vi "main_INA231.vi"() -> ()   [LabVIEW 2011]
uses:
  <vilib>/Utility/file.llb/Read From Spreadsheet File (string).vi
  Global 1.vi
  <vilib>/Utility/file.llb/Write To Spreadsheet File (string).vi
  <vilib>/Utility/file.llb/Write To Spreadsheet File (DBL).vi
panel:
  out "Initial Time":dbl caption="Present (s)"
  out "Selected Path":path
  out "Power History":dbl[](array[numeric])
  out "Current History":dbl[](array[numeric])
  out "Shunt Voltage History":dbl[](array[numeric])
  out "Bus Voltage History":dbl[](array[numeric])
  in  "SM-DIG INT Voltage":enum16{"+3.3V", "+5V"}(ring)
  out "Shunt Voltage":dbl format="%#_4pV"
  out "Bus Voltage":dbl format="%#_4pV"
  out "Power":dbl format="%#_4pW"
  out "Current":dbl format="%#_4pA"
  out "Alert":bool
  out "Conv Ready Flag":bool
  in  "Power":bool=TRUE
  in  "Auto-Write":bool=TRUE
  out "Progress":u8(slide) scale=0.0..100.0
  out "Status":string
  in  "Write All Reg":bool
  in  "Read All Reg":bool
  out "Pending changes \nneed to be written":bool
  in  "Tab Control":T1(tab)
  in  "Enter Current LSB":dbl format="%#_4pA"
  out "High LSB":dbl format="%#_4pA"
  out "Low LSB":dbl format="%#_4pA"
  in  "Config Method":enum16{"Current LSB", "Calibration Register"}(ring)=enum."Calibration Register"
  in  "Enter Value for \nCalibration Register":u16
  in  "Enter Rshunt \nVariables":cluster{"Max Current":dbl, "Resistance":dbl} {"Resistance" format="%#_4p"; "Max Current" format="%#_4pA"}
  in  "Alert Limit":dbl min=0.0 max=0.0 format="%#_4pV"
  in  "Alert Config":T2(ring)=enum."None"
  in  "Conversion Ready":bool
  in  "Shunt Voltage Conversion Time":T3(ring)=enum."1.1ms"
  in  "Bus Voltage Conversion Time":T3(ring)=enum."1.1ms"
  in  "Operating Mode":T4(ring)=enum."Shunt and Bus, Continuous"
  in  "Averaging Mode":T5(ring)
  out "I2C Address":u8 format="%02x"
  in  "A1":u8(ring) items=["GND", "VS+", "SDA", "SCL"]
  in  "A0":u8(ring) items=["GND", "VS+", "SDA", "SCL"]
  out "Shunt Voltage":dbl format="%#_4pV"
  out "Bus Voltage":dbl format="%#_4pV"
  out "Power":dbl format="%#_4pW"
  out "Current":dbl format="%#_4pA"
  out "Current LSB":dbl format="%#_4pA"
  out "Rshunt (Ohms)":dbl format="%#_4p"
  out "Calibration":u16
  out "Shunt Voltage Bin":i16
  out "Current Bin":i16
  out "Power Bin":u16
  out "Bus Voltage Bin":u16
  out "Waveform Graph":dbl[](graph)
  in  "Continuously Poll Data":bool=TRUE
  in  "Graph Config":T6(ring)=enum."Vshunt (V)"
  in  "Help w Reg":bool
  in  "Register Table":i32(listbox)
  in  "dig_bits 16":T7 {"D15" max=1; "D14" max=1; "D13" max=1; "D12" max=1; "D11" max=1; "D10" max=1; "D9" max=1; "D8" max=1 format="%b"; "D7" max=1; "D6" max=1; "D5" max=1; "D4" max=1; "D3" max=1; "D2" max=1; "D1" max=1; "D0" max=1}
  in  "dig_bits8":T8 {"D7" max=1; "D6" max=1; "D5" max=1; "D4" max=1; "D3" max=1; "D2" max=1; "D1" max=1; "D0" max=1}
  out "Bit_Config_16b.csv":path
  out "Start USB DAQ":path
  out "Table_Config.csv":path
  out "USB DAQ INI":path
  out "SAve USB Config":path
  out "Calculate":bool
  out "USB DAQ Vref":dbl min=0.0 max=5.0
  out "USB DAQ Address":i32 format="%x"
  out "DAC Mode":i32
  out "ADS Mode":i32
  out "USB DAQ Vsup":dbl min=0.0 max=5.0
  in  "Register":u16[](array[numeric]) format="%x"
  out "bit_text_array":string[][](array[string])=[["d0", "d1", "d2", "d3", "d4", "d5", "d6", "d7"], ["a0", "a1", "a2", "a3", "a4", "a5", "a6", "a7"]]
  out "Digital out":u16
  out "Reg_Numb":i32
  out "Number of Registers":i32
  in  "PORT2":i16=152 format="%x"
  out "Numb_Bits_In_Reg":i32=16
  out "Edited Register":bool[](array[boolean])
  out "Index to Reg No":u8[](array[numeric]) format="%x"
  out "Alert Limit Digital":i16
  in  "Write I2C Address":u8 format="%x"
  out "RAR trigger":bool
  out "1st Time?":bool
  # "Step 4: Select Configuration Method"
  # "Step 5: Set Configuration Register"
  # "Current LSB"
  # "Step 6: Configure Alert Pin"
  # "Step 3: Set Conversion Times"
  # "Bus Conversion"
  # "Shunt Conversion"
  # "Step 2: Configure Operation"
  # "Step 1: Set I2C Address"
  # "This tab gives a flow chart of how the calculations within the INA226 occur"
  # "Current * Bus Voltage"
  # "__________________"
  # "Power ="
  # "20000"
  # "Shunt Voltage * Cal"
  # "________________"
  # "Current ="
  # "2048"
  # ".00512"
  # "_________________"
  # "Cal ="
  # "Current LSB *Rshunt"
  # "20000"
  # "÷"
  # "2048"
  # "÷"
  # ".00512"
  # "÷"
  # "X"
  # "X"
  # "X"
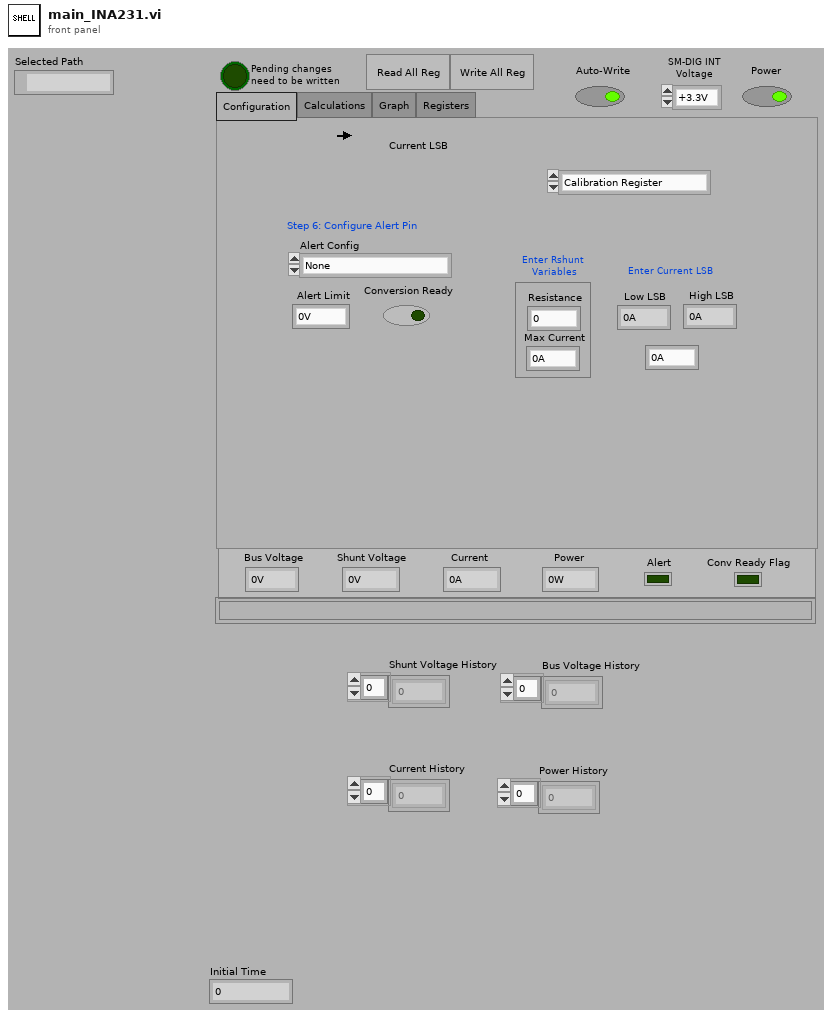
[diagram p1: front panel]
types:
  T1 = enum32{"Configuration", "Calculations", "Graph", "Registers", "Debug", "Internal Variables"}
  T2 = enum16{"Over-Limit Power", "Bus Voltage Under-Voltage", "Bus Voltage Over-Voltage", "Shunt Voltage Under-Voltage", "Shunt Voltage Over-Voltage", "None"}
  T3 = enum16{"140us", "204us", "332us", "588us", "1.1ms", "2.116ms", "4.156ms", "8.244ms"}
  T4 = enum16{"Power Down", "Shunt Voltage, Triggered", "Bus Voltage, Triggered", "Shunt and Bus, Triggered", "Power Down ", "Shunt Voltage, Continuous", "Bus Voltage, Continuous", "Shunt and Bus, Continuous"}
  T5 = enum16{"1", "4", "16", "64", "128", "256", "512", "1024"}
  T6 = enum16{"Vbus (V)", "Vshunt (V)", "Current (A)", "Power (W)"}
  T7 = cluster{"D0":u16, "D1":u16, "D2":u16, "D3":u16, "D4":u16, "D5":u16, "D6":u16, "D7":u16, "D8":u16, "D9":u16, "D10":u16, "D11":u16, "D12":u16, "D13":u16, "D14":u16, "D15":u16}
  T8 = cluster{"D0":u16, "D1":u16, "D2":u16, "D3":u16, "D4":u16, "D5":u16, "D6":u16, "D7":u16}
  T9 = enum16{"Always On", "Always Off", "Off While Running"}
  T10 = enum32{"Invalid", "Standard", "Closed", "Hidden", "Minimized", "Maximized"}
  T11 = enum16{"Over-Limit Power", "Bus Voltage Under-Voltage", "Bus Voltage Over-Voltage", "Shunt Voltage Under-Voltage", "Shunt Voltage Over-Voltage"}
  T12 = enum32{"invalid app kind", "Development System", "Run Time System", "Student Edition", "Embedded LabVIEW", "Evaluation", "Custom"}
  T13 = typedef "LVRowAndColumnTypeDef.ctl" = cluster{"Row":i32, "Column":i32}
  T14 = cluster{"[0]":u16, "[1]":u16, "[2]":u16, "[3]":u16, "[4]":u16, "[5]":u16, "[6]":u16, "[7]":u16}
  T15 = cluster{"[0]":u16, "[1]":u16, "[2]":u16, "[3]":u16, "[4]":u16, "[5]":u16, "[6]":u16, "[7]":u16, "[8]":u16, "[9]":u16, "[10]":u16, "[11]":u16, "[12]":u16, "[13]":u16, "[14]":u16, "[15]":u16}
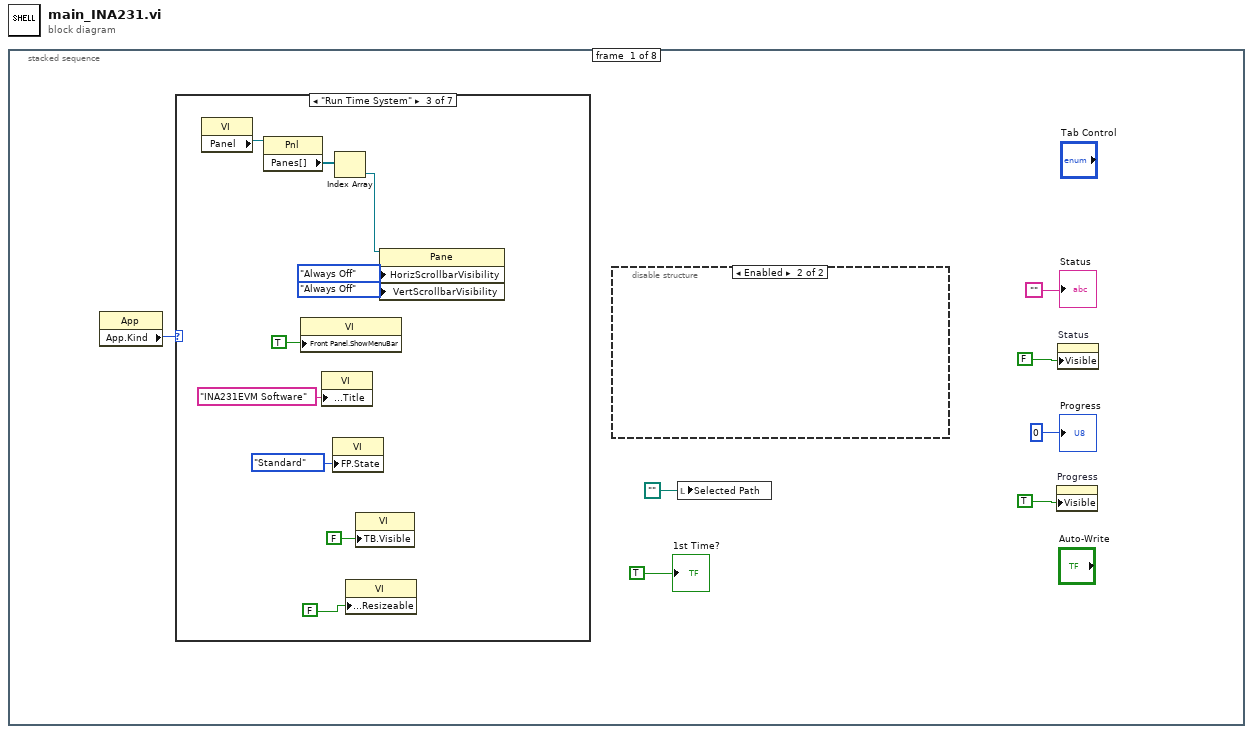
[diagram p0: block diagram]
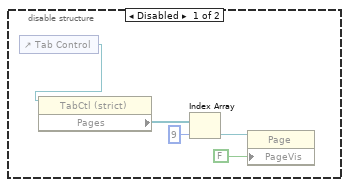
[diagram p2: hidden frame]
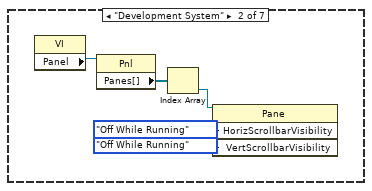
[diagram p4: hidden frame]
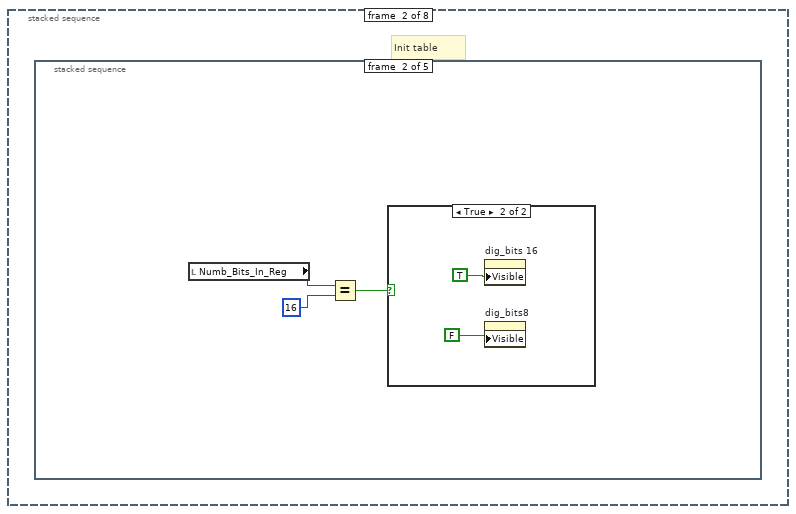
[diagram p9: hidden frame]
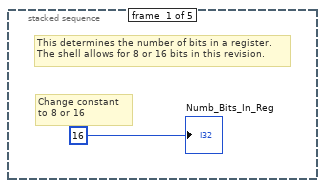
[diagram p10: hidden frame]
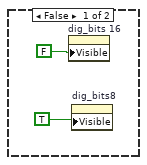
[diagram p11: hidden frame]
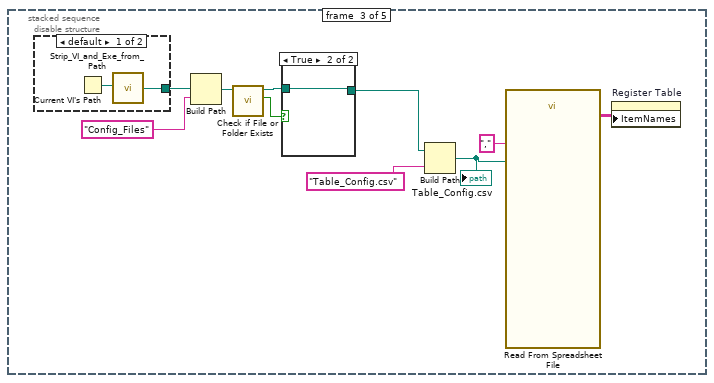
[diagram p12: hidden frame]
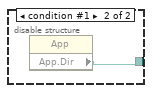
[diagram p13: hidden frame]
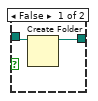
[diagram p14: hidden frame]
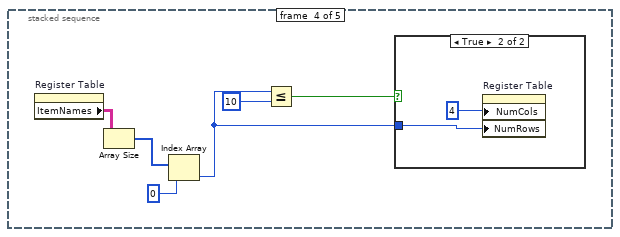
[diagram p15: hidden frame]
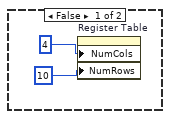
[diagram p16: hidden frame]
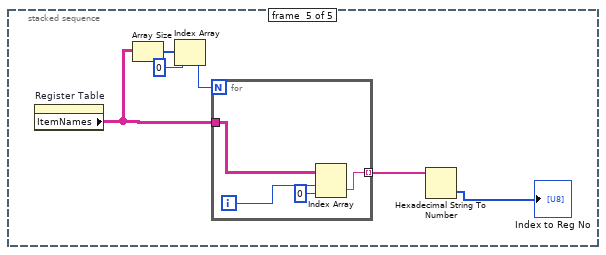
[diagram p17: hidden frame]
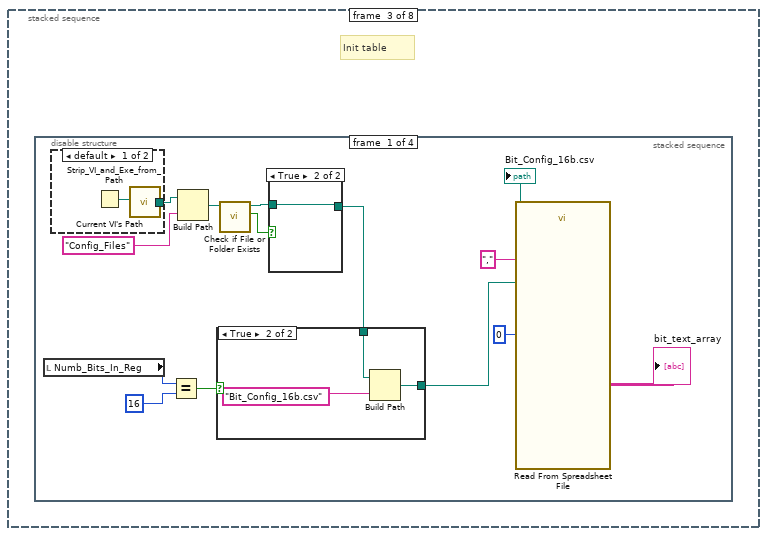
[diagram p18: hidden frame]
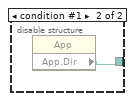
[diagram p19: hidden frame]
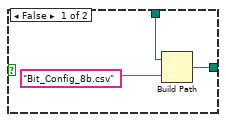
[diagram p20: hidden frame]
diagram:
  n1 = stacked-sequence {
    frame #0 {
      n2 = property class="App"() -> ("App.Kind"=w7:T12)  [unwired: 2 in, 2 out]
      n3 = case shown="\"Run Time System\"" w7 {
        frame "invalid app kind", Default {
        }
        frame "Development System" {
          n4 = property class="VI"() -> ("Panel"=w17:refnum<vi>)  [unwired: 2 in, 2 out]
          n5 = property class="Pnl"(reference=w17) -> ("Panes[]"=w16:refnum<vi>[])  [unwired: 1 in, 2 out]
          n6 = Index Array(array=w16) -> (element=w15:refnum<vi>)  [unwired: 1 in]
          n7 = property class="Pane"(reference=w15, "HorizScrollbarVisibility"=T9."Off While Running" ("Horizontal Scrollbar Visibility"), "VertScrollbarVisibility"=T9."Off While Running" ("Vertical Scrollbar Visibility")) -> ()  [unwired: 1 in, 2 out]
        }
        frame "Run Time System" {
          n8 = property class="VI"() -> ("Panel"=w27:refnum<vi>)  [unwired: 2 in, 2 out]
          n9 = property class="Pnl"(reference=w27) -> ("Panes[]"=w26:refnum<vi>[])  [unwired: 1 in, 2 out]
          n10 = property class="VI"("Front Panel.ShowMenuBar"=TRUE ("Front Panel Window:Show Menu Bar")) -> ()  [unwired: 2 in, 2 out]
          n11 = property class="VI"("Front Panel.Title"="INA231EVM Software" ("Front Panel Window:Title")) -> ()  [unwired: 2 in, 2 out]
          n12 = property class="VI"("FP.State"=T10."Standard" ("Front Panel Window:State")) -> ()  [unwired: 2 in, 2 out]
          n13 = Index Array(array=w26) -> (element=w25:refnum<vi>)  [unwired: 1 in]
          n14 = property class="VI"("Front Panel.Resizeable"=FALSE ("Front Panel Window:Resizeable")) -> ()  [unwired: 2 in, 2 out]
          n15 = property class="VI"("TB.Visible"=FALSE ("Front Panel Window:Resizeable")) -> ()  [unwired: 2 in, 2 out]
          n16 = property class="Pane"(reference=w25, "HorizScrollbarVisibility"=T9."Always Off" ("Horizontal Scrollbar Visibility"), "VertScrollbarVisibility"=T9."Always Off" ("Vertical Scrollbar Visibility")) -> ()  [unwired: 1 in, 2 out]
        }
        frame "Student Edition" {
        }
        frame "Embedded LabVIEW" {
        }
        frame "Evaluation" {
        }
        frame "Custom" {
        }
      }
      n17 = disable-structure shown="Enabled" {
        frame Disabled {
          n18 = control-ref of="Tab Control"() -> (w8:refnum<vi>)
          n19 = property class="TabCtl (strict)"(reference=w8) -> ("Pages"=w11:refnum<vi>[])  [unwired: 1 in, 2 out]
          n20 = Index Array(array=w11, index=9) -> (element=w9:refnum<vi>)
          n21 = property class="Page"(reference=w9, "PageVis"=FALSE ("Page Visible")) -> ()  [unwired: 1 in, 2 out]
        }
        frame Enabled {
        }
      }
      n22 = local write "Selected Path"(path "") -> ()
      n23 = property on="Progress" class="Slide (strict)"("Visible"=TRUE ("Front Panel Window:Resizeable")) -> ()  [unwired: 2 in, 2 out]
      n24 = property on="Status" class="Str"("Visible"=FALSE ("Front Panel Window:Resizeable")) -> ()  [unwired: 2 in, 2 out]
      "Progress" <- u8 0 ("Progress")
      "Status" <- ""
      "1st Time?" <- TRUE ("1st Time?")
    }
    frame #1 {
      # "Init table"
      n25 = stacked-sequence {
        frame #0 {
          # "Change constant \nto 8 or 16"
          # "This determines the number of bits in a register.\nThe shell allows for 8 or 16 bits in this revision."
          "Numb_Bits_In_Reg" <- 16
        }
        frame #1 {
          n26 = local read "Numb_Bits_In_Reg"() -> (w31:i32)
          n27 = Equal?(x=w31, y=16) -> (x = y?=w30:bool)
          n28 = case shown="True" w30 {
            frame False {
              n29 = property on="dig_bits 16" class="Clust (strict)"("Visible"=FALSE) -> ()  [unwired: 2 in, 2 out]
              n30 = property on="dig_bits8" class="Clust (strict)"("Visible"=TRUE) -> ()  [unwired: 2 in, 2 out]
            }
            frame True {
              n31 = property on="dig_bits 16" class="Clust (strict)"("Visible"=TRUE) -> ()  [unwired: 2 in, 2 out]
              n32 = property on="dig_bits8" class="Clust (strict)"("Visible"=FALSE) -> ()  [unwired: 2 in, 2 out]
            }
          }
        }
        frame #2 {
          n33 = disable-structure shown="default" {
            disable-tunnel: [w46 w48] -> w44
            frame condition #0 (active) {
              n34 = Current VI's Path() -> (path=w47:path)
              n35 = call "Strip_VI_and_Exe_from_Path.vi"("App Path"=w47) -> ("App Path out"=w46:path)
            }
            frame condition #1 {
              n36 = property class="App"() -> ("App.Dir"=w48:path)  [unwired: 2 in, 2 out]
            }
          }
          n37 = Build Path(base path=w44, name or relative path="Config_Files" ("path name")) -> (appended path=w43:path)
          n38 = call <vilib>:"Check if File or Folder Exists.vi"("path"=w43) -> ("file or folder exists?"=w42:bool, "dup path"=w41:path)  [unwired: 8 in, 1 out]
          n39 = case shown="True" w42 {
            tunnel: w41 -> [w50 w51]
            tunnel: [w49 w51] -> w38
            frame False {
              n40 = Create Folder(path (use dialog)=w50) -> (created path=w49:path)  [unwired: 2 in, 2 out]
            }
            frame True {
            }
          }
          n41 = Build Path(base path=w38, name or relative path="Table_Config.csv") -> (appended path=w45:path)
          "Table_Config.csv" <- w45
          n42 = call-poly <vilib>:"Read From Spreadsheet File.vi"("delimiter (\\t)"="," ("delimiter (\\t)"), "file path (dialog if empty)"=w45) -> ("all rows"=w37:string[][])  [unwired: 5 in, 4 out]
          n43 = property on="Register Table" class="MCListbox (strict)"("ItemNames"=w37) -> ()  [unwired: 2 in, 2 out]
        }
        frame #3 {
          n44 = property on="Register Table" class="MCListbox (strict)"() -> ("ItemNames"=w52:string[][])  [unwired: 2 in, 2 out]
          n45 = Array Size(array=w52) -> (size(s)=w53:i32[])
          n46 = Index Array(array=w53, index=0) -> (element=w57:i32)
          n47 = Less Or Equal?(x=w57, y=10) -> (x <= y?=w55:bool)
          n48 = case shown="True" w55 {
            tunnel: w57 -> [_ w60]
            frame False {
              n49 = property on="Register Table" class="MCListbox (strict)"("NumCols"=u32 4 ("Number of Columns"), "NumRows"=u32 10 ("Number of Rows")) -> ()  [unwired: 2 in, 2 out]
            }
            frame True {
              n50 = property on="Register Table" class="MCListbox (strict)"("NumCols"=u32 4 ("Number of Columns"), "NumRows"=w60) -> ()  [unwired: 2 in, 2 out]
            }
          }
        }
        frame #4 {
          n51 = property on="Register Table" class="MCListbox (strict)"() -> ("ItemNames"=w63:string[][])  [unwired: 2 in, 2 out]
          n52 = Array Size(array=w63) -> (size(s)=w65:i32[])
          n53 = Index Array(array=w65, index=0) -> (element=w67:i32)
          n54 = for {
            N: w67 -> [_]
            tunnel: w63 -> [w70]
            tunnel: [w68] -> w64 mode=indexing
            i -> [w71]
            n55 = Index Array(array=w70, index (row)=w71, index (col)=0 ("disabled index (col)")) -> (element=w68:string)
          }
          n56 = Hexadecimal String To Number(string=w64) -> (number=→"Index to Reg No":u32[])  [unwired: 2 in, 1 out]
        }
      }
    }
    frame #2 {
      # "Init table"
      n57 = stacked-sequence {
        frame #0 {
          n58 = local read "Numb_Bits_In_Reg"() -> (w74:i32)
          n59 = disable-structure shown="default" {
            disable-tunnel: [w85 w87] -> w72
            frame condition #0 (active) {
              n60 = Current VI's Path() -> (path=w86:path)
              n61 = call "Strip_VI_and_Exe_from_Path.vi"("App Path"=w86) -> ("App Path out"=w85:path)
            }
            frame condition #1 {
              n62 = property class="App"() -> ("App.Dir"=w87:path)  [unwired: 2 in, 2 out]
            }
          }
          n63 = Equal?(x=w74, y=16) -> (x = y?=w75:bool)
          n64 = Build Path(base path=w72, name or relative path="Config_Files" ("path name")) -> (appended path=w83:path)
          n65 = call <vilib>:"Check if File or Folder Exists.vi"("path"=w83) -> ("file or folder exists?"=w82:bool, "dup path"=w81:path)  [unwired: 8 in, 1 out]
          n66 = case shown="True" w82 {
            tunnel: w81 -> [w95 w96]
            tunnel: [w94 w96] -> w79
            frame False {
              n67 = Create Folder(path (use dialog)=w95) -> (created path=w94:path)  [unwired: 2 in, 2 out]
            }
            frame True {
            }
          }
          n68 = case shown="True" w75 {
            tunnel: [w88 w93] -> w84
            tunnel: w79 -> [w89 w91]
            frame False {
              n69 = Build Path(base path=w89, name or relative path="Bit_Config_8b.csv") -> (appended path=w88:path)
            }
            frame True {
              n70 = Build Path(base path=w91, name or relative path="Bit_Config_16b.csv") -> (appended path=w93:path)
            }
          }
          "Bit_Config_16b.csv" <- w84
          n71 = call-poly <vilib>:"Read From Spreadsheet File.vi"("delimiter (\\t)"="," ("delimiter (\\t)"), "start of read offset (chars.:0)"=0, "file path (dialog if empty)"=w84) -> ("all rows"=→"bit_text_array":string[][])  [unwired: 4 in, 4 out]
        }
        frame #1 {
          n72 = property on="Register Table" class="MCListbox (strict)"() -> ("ItemNames"=w104:string[][])  [unwired: 2 in, 2 out]
          n73 = local read "bit_text_array"() -> (w99:string[][])
          n74 = Array Size(array=w104) -> (size(s)=w103:i32[])
          n75 = Index Array(array=w103, index=0) -> (element=w105:i32)
          n76 = Array Size(array=w99) -> (size(s)=w98:i32[])
          n77 = Index Array(array=w98, index=0) -> (element=w97:i32)
          n78 = Not Equal?(x=w105, y=w97) -> (x != y?=w101:bool)
          n79 = case shown="True" w101 {
            frame False {
            }
            frame True {
              n80 = One Button Dialog(message="The number of rows in \"Bit_Config.csv\"  is not \nequal to the number of rows in \"Table_Config.csv\"" ("button name (\"OK\")")) -> ()  [unwired: 1 in, 1 out]
            }
          }
        }
        frame #2 {
          # "init table rows and col"
          n81 = property on="Register Table" class="MCListbox (strict)"("ColHdrString"=string[] ["Addr", "Name", "Status", "Hex", "Value"] ("Column Header Strings[]")) -> ()  [unwired: 2 in, 2 out]
        }
        frame #3 {
          n82 = local write "Pending changes \nneed to be written"(FALSE ("Pending changes \nneed to be written")) -> ()
          n83 = local read "bit_text_array"() -> (w115:string[][])
          n84 = Array Size(array=w115) -> (size(s)=w114:i32[])
          n85 = Index Array(array=w114, index=0) -> (element=w109:i32)
          "Number of Registers" <- w109
          n86 = Initialize Array(FALSE ("Boolean"), w109) -> (→"Edited Register":bool[])
          n87 = Initialize Array(0 ("element"), w109) -> (w108:i32[])
          n88 = local write "Register"(w108) -> ()
          n89 = disable-structure shown="Disabled" {
            frame Disabled {
              n90 = property on="Register" class="Arr (strict)" props=["Val(Sgnl)"]() -> ()  [unwired: 3 in, 2 out]
            }
            frame Enabled {
            }
          }
        }
      }
    }
    frame #3 {
      n91 = Current VI's Path() -> (path=w122:path)
      n92 = call "Load_USB_DAQ_Config_File.vi"("App Path"=w122) -> ("USB DAQ Vsup"=→"USB DAQ Vsup":dbl, "USB DAQ Address"=→"USB DAQ Address":i32, "DAC Mode"=→"DAC Mode":i32, "ADS Mode"=→"ADS Mode":i32, "USB DAQ Vref"=→"USB DAQ Vref":dbl)
    }
    frame #4 {
      n93 = flat-sequence {
        frame #0 {
          n94 = call "TI_INIT.vi"() -> ()  [unwired: 1 in, 2 out]
        }
        frame #1 {
          n95 = local read "USB DAQ Address"() -> (w126:i32)
          n96 = Current VI's Path() -> (path=w125:path)
          "Start USB DAQ" <- w125
          n97 = call "Start_USB_DAQ.vi"("USB ADDRESS In"=w126, "App Path"=w125) -> ("Abort"=w124:bool, "USB ADDRESS 0ut"=w123:i32)
          n98 = local write "USB DAQ Address"(w123) -> ()
          n99 = Stop(stop? (T)=w124) -> ()
        }
        frame #2 {
          # "Power on for typical starting conditions"
          n100 = local read "USB DAQ Address"() -> (w128:i32)
          n101 = local write "PORT2"(i16 152 ("PORT2")) -> ()
          n102 = call "VDUT ON.vi"("Device address"=w128) -> ()  [unwired: 2 in, 1 out]
        }
      }
    }
    frame #5 {
      w132 = dbl[] [] ("History Data")
      w141 = 0.0 ("Power")
      w146 = 0.0 ("Power")
      w140 = FALSE
      n103 = local read "Enter Rshunt \nVariables"() -> (w142:cluster{"Max Current":dbl, "Resistance":dbl})
      n104 = local write "I2C Address"(w141) -> ()
      n105 = Bundle By Name(cluster=w142, "Max Current"=w141, "Resistance"=w141) -> (w143:cluster{"Max Current":dbl, "Resistance":dbl})
      n106 = local write "Enter Rshunt \nVariables"(w143) -> ()
      n107 = local write "Config Method"(enum16{"Current LSB", "Calibration Register"}."Current LSB" ("Config Method")) -> ()
      n108 = local write "Operating Mode"(T4."Shunt Voltage, Continuous" ("Operating Mode")) -> ()
      n109 = local write "Shunt Voltage Conversion Time"(T3."1.1ms" ("Shunt Voltage Conversion Time")) -> ()
      n110 = local write "Bus Voltage Conversion Time"(T3."1.1ms" ("Bus Voltage Conversion Time")) -> ()
      n111 = local write "Alert Config"(T2."None" ("Alert Config")) -> ()
      n112 = local write "Alert Limit"(w141) -> ()
      n113 = local write "A0"(w141) -> ()
      n114 = local write "Write I2C Address"(u8 128 ("Write I2C Address")) -> ()
      n115 = local write "A1"(w141) -> ()
      n116 = local write "Averaging Mode"(w141) -> ()
      n117 = local write "Enter Value for \nCalibration Register"(w146) -> ()
      n118 = local write "Enter Current LSB"(w146) -> ()
      n119 = local write "High LSB"(w146) -> ()
      n120 = local write "Low LSB"(w146) -> ()
      n121 = local write "Shunt Voltage"(w146) -> ()
      n122 = local write "Continuously Poll Data"(w140) -> ()
      n123 = local write "Current"(w146) -> ()
      n124 = local write "Conversion Ready"(w140) -> ()
      n125 = local write "Bus Voltage"(w146) -> ()
      n126 = local write "Alert"(w140) -> ()
      n127 = local write "Conv Ready Flag"(w140) -> ()
      n128 = local write "Power"(w146) -> ()
      n129 = local write "Graph Config"(T6."Vbus (V)" ("Graph Config")) -> ()
      n130 = global read "Global 1.vi" "SAve USB Config"() -> (→"SAve USB Config":path)
      n131 = global read "Global 1.vi" "USB DAQ INI"() -> (→"USB DAQ INI":path)
      n132 = property on="Enter Value for \nCalibration Register" class="DigNum (strict)"("Visible"=FALSE) -> ()  [unwired: 2 in, 2 out]
      n133 = property on="Max Current" class="DigNum (strict)"("Visible"=TRUE) -> ()  [unwired: 2 in, 2 out]
      n134 = property on="Enter Current LSB" class="DigNum (strict)"("Visible"=TRUE) -> ()  [unwired: 2 in, 2 out]
      n135 = property on="Low LSB" class="DigNum (strict)"("Visible"=TRUE) -> ()  [unwired: 2 in, 2 out]
      n136 = property on="High LSB" class="DigNum (strict)"("Visible"=TRUE) -> ()  [unwired: 2 in, 2 out]
      n137 = local write "Shunt Voltage History"(w132) -> ()
      n138 = local write "Current History"(w132) -> ()
      n139 = local write "Bus Voltage History"(w132) -> ()
      n140 = local write "Power History"(w132) -> ()
      n141 = local write "Waveform Graph"(w132) -> ()
    }
    frame #6 {
      n142 = property on="RAR trigger" class="Bool (strict)"("Val(Sgnl)"=TRUE) -> ()  [unwired: 2 in, 2 out]
    }
    frame #7 {
      n143 = while {
        stop <- w151 stop-if-true
        n144 = event shown="[2] Menu Selection (User)" {
          selector: _ -> [_ _ _ _ _ _ _ _ _ _ _ _ _ _ _ _ _ _ _ _ _ _ _ _ _ _ _ _ _]
          dyn-events: _ -> [_ _ _ _ _ _ _ _ _ _ _ _ _ _ _ _ _ _ _ _ _ _ _ _ _ _ _ _ _]
          timeout: 800 -> [_ _ _ _ _ _ _ _ _ _ _ _ _ _ _ _ _ _ _ _ _ _ _ _ _ _ _ _ _]
          tunnel: [_ _ _ w233 _ _ _ _ _ _ _ _ _ _ _ _ _ _ _ _ _ _ _ _ _ _ _ _ _] -> w151
          event Timeout {
            n145 = event-data() -> ()  [unwired: 1 in, 2 out]
            n146 = case shown="True" "Continuously Poll Data" {
              frame False {
                n147 = property on="Write All Reg" class="Bool"() -> ("Disabled"=w153:u8)  [unwired: 2 in, 2 out]
                n148 = case shown="0, Default" w153 {
                  frame 0, Default {
                  }
                  frame 1 {
                  }
                  frame 2 {
                    n149 = property on="Write All Reg" class="Bool"("Disabled"=u8 0) -> ()  [unwired: 2 in, 2 out]
                  }
                }
              }
              frame True {
                n150 = stacked-sequence {
                  frame #0 {
                    n151 = local read "1st Time?"() -> (w155:bool)
                    n152 = case shown="True" w155 {
                      frame False {
                      }
                      frame True {
                        n153 = call "Elapsed Time"() -> ("Present (s)"=w157:dbl)  [unwired: 12 in, 7 out]
                        n154 = local write "Initial Time"(w157) -> ()
                        n155 = local write "1st Time?"(FALSE ("1st Time?")) -> ()
                      }
                    }
                  }
                  frame #1 {
                    n156 = property on="Write All Reg" class="Bool"("Disabled"=u8 2) -> ()  [unwired: 2 in, 2 out]
                    n157 = property on="RAR trigger" class="Bool (strict)"("Val(Sgnl)"=TRUE) -> ()  [unwired: 2 in, 2 out]
                  }
                }
              }
            }
          }
          event "Graph Config": Value Change {
            n158 = event-data() -> ()  [unwired: 1 in, 6 out]
            n159 = case shown="\"Current (A)\"" "Graph Config" {
              frame "Vbus (V)", Default {
                n160 = local read "Bus Voltage History"() -> (w161:dbl[])
                n161 = local write "Waveform Graph"(w161) -> ()
              }
              frame "Vshunt (V)" {
                n162 = local read "Shunt Voltage History"() -> (w162:dbl[])
                n163 = local write "Waveform Graph"(w162) -> ()
              }
              frame "Current (A)" {
                n164 = local read "Current History"() -> (w163:dbl[])
                n165 = local write "Waveform Graph"(w163) -> ()
              }
              frame "Power (W)" {
                n166 = local read "Power History"() -> (w164:dbl[])
                n167 = local write "Waveform Graph"(w164) -> ()
              }
            }
          }
          event Menu Selection (User) {
            n168 = event-data() -> ("MenuRef"=w165:refnum<k9>, "ItemTag"=w166:string)  [unwired: 1 in, 5 out]
            n169 = stacked-sequence {
              tunnel: w166 -> [w169 w173 w178 w183 w186 _]
              tunnel: w166 -> [_ _ _ _ _ w216]
              tunnel: w165 -> [_ _ _ _ w185 _]
              frame #0 {
                n170 = Equal?(x=w169, y="Control / Measure Bits") -> (x = y?=w168:bool)
                n171 = case shown="True" w168 {
                  frame False {
                  }
                  frame True {
                    n172 = local read "USB DAQ Address"() -> (w170:i32)
                    n173 = call "GPIO_Control.vi"("Device address"=w170) -> ()
                  }
                }
              }
              frame #1 {
                n174 = Equal?(x=w173, y="DAC / ADC Control") -> (x = y?=w171:bool)
                n175 = case shown="True" w171 {
                  frame False {
                  }
                  frame True {
                    n176 = local read "USB DAQ Address"() -> (w174:i32)
                    n177 = local read "ADS Mode"() -> (w176:i32)
                    n178 = call "ADC_and_DAC.vi"("ADS Mode In"=w176, "Board address"=w174) -> ("ADS Mode Out"=w175:i32)
                    n179 = local write "ADS Mode"(w175) -> ()
                  }
                }
              }
              frame #2 {
                n180 = Equal?(x=w178, y="Run Mnemonic Commands") -> (x = y?=w179:bool)
                n181 = case shown="True" w179 {
                  frame False {
                  }
                  frame True {
                    n182 = local read "USB DAQ Address"() -> (w180:i32)
                    n183 = call "Run_4_Cmds.vi"("USB DAQ Address"=w180) -> ()  [unwired: 2 in]
                  }
                }
              }
              frame #3 {
                n184 = Equal?(x=w183, y="Debug") -> (x = y?=w181:bool)
                n185 = case shown="False" w181 {
                  frame False {
                  }
                  frame True {
                    n186 = call "TI_Debug_Window.vi"() -> ()  [unwired: 1 in]
                  }
                }
              }
              frame #4 {
                w184 = "Make All Visible" ("y")
                n187 = Equal?(x=w186, y=w184) -> (x = y?=w187:bool)
                n188 = case shown="True" w187 {
                  tunnel: w185 -> [_ w189]
                  tunnel: w184 -> [_ w190]
                  frame False {
                  }
                  frame True {
                    n189 = Get Menu Item Info(7:w190, 11:w189) -> (3:w188:refnum<k9>, 4:w191:bool)  [unwired: 1 in, 5 out]
                    n190 = case shown="False" w191 {
                      tunnel: w190 -> [w193 w205]
                      tunnel: w188 -> [w192 w204]
                      frame True {
                        n191 = stacked-sequence {
                          tunnel: w193 -> [_ _ w202]
                          tunnel: w192 -> [_ _ w201]
                          frame #0 {
                            n192 = control-ref of="Tab Control"() -> (w194:refnum<vi>)
                            n193 = property class="TabCtl (strict)"(reference=w194) -> ("Pages"=w197:refnum<vi>[])  [unwired: 1 in, 2 out]
                            n194 = Index Array(array=w197, index=4) -> (element=w195:refnum<vi>)
                            n195 = property class="Page"(reference=w195, "PageVis"=FALSE ("Page Visible")) -> ()  [unwired: 1 in, 2 out]
                          }
                          frame #1 {
                            n196 = property on="Status" class="Str"("Visible"=TRUE ("Page Visible")) -> ()  [unwired: 2 in, 2 out]
                            n197 = property on="Progress" class="Slide (strict)"("Visible"=TRUE) -> ()  [unwired: 2 in, 2 out]
                          }
                          frame #2 {
                            n198 = Set Menu Item Info(6:FALSE ("checked"), 7:w202, 11:w201) -> ()  [unwired: 4 in, 2 out]
                          }
                        }
                      }
                      frame False {
                        n199 = stacked-sequence {
                          tunnel: w205 -> [_ _ w214]
                          tunnel: w204 -> [_ _ w213]
                          frame #0 {
                            n200 = control-ref of="Tab Control"() -> (w206:refnum<vi>)
                            n201 = property class="TabCtl (strict)"(reference=w206) -> ("Pages"=w209:refnum<vi>[])  [unwired: 1 in, 2 out]
                            n202 = Index Array(array=w209, index=4) -> (element=w207:refnum<vi>)
                            n203 = property class="Page"(reference=w207, "PageVis"=TRUE ("Page Visible")) -> ()  [unwired: 1 in, 2 out]
                          }
                          frame #1 {
                            n204 = property on="Status" class="Str"("Visible"=TRUE ("Page Visible")) -> ()  [unwired: 2 in, 2 out]
                            n205 = property on="Progress" class="Slide (strict)"("Visible"=TRUE) -> ()  [unwired: 2 in, 2 out]
                          }
                          frame #2 {
                            n206 = Set Menu Item Info(6:TRUE ("checked"), 7:w214, 11:w213) -> ()  [unwired: 4 in, 2 out]
                          }
                        }
                      }
                    }
                  }
                }
              }
              frame #5 {
                n207 = Equal?(x=w216, y="Start Graph Log") -> (x = y?=w217:bool)
                n208 = case shown="True" w217 {
                  frame False {
                  }
                  frame True {
                    n209 = Current VI's Path() -> (path=w226:path)
                    n210 = call "Open_File_from_Folder.vi"("path name"="Output Data", "prompt"="Save Config File", "pattern label"="CSV File ", "pattern (all files)"="*.csv", "App Path"=w226) -> ("selected path"=w220:path, "cancelled"=w221:bool)
                    n211 = local write "1st Time?"(TRUE ("1st Time?")) -> ()
                    n212 = case shown="False" w221 {
                      tunnel: w220 -> [w227 _]
                      frame False {
                        n213 = call-poly <vilib>:"Write To Spreadsheet File.vi"("delimiter (\\t)"="," ("delimiter (\\t)"), "append to file? (new file:F)"=TRUE, "1D data"=string[] ["Time", "Vbus", "Vshunt", "Current", "Power"], "file path (dialog if empty)"=w227) -> ()  [unwired: 4 in, 1 out]
                        "Selected Path" <- w227
                      }
                      frame True {
                        n214 = local write "Selected Path"(path "") -> ()
                      }
                    }
                  }
                }
              }
            }
          }
          event Panel Close? {
            n215 = event-data() -> ()  [unwired: 1 in, 4 out]
            n216 = flat-sequence {
              tunnel: [w237] -> w232
              tunnel: [w239] -> w233
              tunnel: w232 -> [w239]
              frame #0 {
                n217 = Two Button Dialog(message="Are you sure that you want to close this application?", 1:"No" ("F button name (\"Cancel\")"), 2:"Yes" ("T button name (\"OK\")")) -> (T button?=w237:bool)
              }
              frame #1 {
                n218 = case shown="True" w239 {
                  frame False {
                  }
                  frame True {
                    n219 = call "tio32_Close.vi"() -> ()  [unwired: 6 in, 3 out]
                  }
                }
              }
            }
            n220 = Not(x=w233) -> (.not. x?=w234:bool)
            n221 = event-data("Discard?"=w234) -> ()  [unwired: 1 in, 1 out]
          }
          event "SM-DIG INT Voltage": Value Change {
            n222 = event-data() -> ()  [unwired: 1 in, 6 out]
            n223 = case shown="\"+3.3V\", Default" "SM-DIG INT Voltage" {
              frame "+3.3V", Default {
                n224 = local read "PORT2"() -> (w241:i16)
                n225 = call "SM_VDUT SEL.vi"("Port2 IN"=w241, "Power Voltage"=enum16{"+3.3V", "+5V"}."+3.3V") -> ("Port2 OUT"=w242:u8)  [unwired: 1 in, 1 out]
                n226 = local write "PORT2"(w242) -> ()
              }
              frame "+5V" {
                n227 = local read "PORT2"() -> (w244:i16)
                n228 = call "SM_VDUT SEL.vi"("Port2 IN"=w244, "Power Voltage"=enum16{"+3.3V", "+5V"}."+5V") -> ("Port2 OUT"=w245:u8)  [unwired: 1 in, 1 out]
                n229 = local write "PORT2"(w245) -> ()
              }
            }
          }
          event "dig_bits 16", "dig_bits8": Value Change {
            n230 = event-data() -> ()  [unwired: 1 in, 6 out]
            n231 = stacked-sequence {
              frame #0 {
                n232 = local write "Digital out"(u16 0 ("Digital out")) -> ()
              }
              frame #1 {
                # "Converts the cluster of bits to a decimal equivelant."
                n233 = local read "Numb_Bits_In_Reg"() -> (w251:i32)
                n234 = Equal?(x=w251, y=16) -> (x = y?=w249:bool)
                n235 = case shown="True" w249 {
                  tunnel: [w252 w255] -> w248
                  frame False {
                    n236 = Cluster To Array(cluster="dig_bits8") -> (array=w252:u16[])
                  }
                  frame True {
                    n237 = Cluster To Array(cluster="dig_bits 16") -> (array=w255:u16[])
                  }
                }
                n238 = for {
                  tunnel: w248 -> [w258] mode=indexing
                  i -> [w257]
                  n239 = local read "Digital out"() -> (w259:u16)
                  n240 = Logical Shift(y=w257, x=w258) -> (x << y=w260:u16)
                  n241 = Add(x=w260, y=w259) -> (x+y=→"Digital out":u16)
                }
              }
              frame #2 {
                # "Takes the decimal equivelant from the bit cluster and places\n it into the list box."
                n242 = local read "Numb_Bits_In_Reg"() -> (w266:i32)
                n243 = local read "Digital out"() -> (w269:u16)
                n244 = Number To Hexadecimal String(1:i16 2 ("width (-)"), 2:w269) -> (0:w263:string)
                n245 = local read "Reg_Numb"() -> (w271:i32)
                n246 = Equal?(x=w266, y=8) -> (x = y?=w264:bool)
                n247 = property on="Register Table" class="MCListbox (strict)"() -> ("ItemNames"=w268:string[][])  [unwired: 2 in, 2 out]
                n248 = case shown="False" w264 {
                  tunnel: w263 -> [w272 w274]
                  tunnel: [w272 w273] -> w262
                  frame False {
                  }
                  frame True {
                    n249 = String Subset(string=w274, length (rest)=2 ("length (rest)")) -> (substring=w273:string)  [unwired: 1 in]
                  }
                }
                n250 = Replace Array Subset(array=w268, new element=w262, index (row)=w271, index (col)=3 ("disabled index (col)")) -> (w267:string[][])
                n251 = property on="Register Table" class="MCListbox (strict)"("ItemNames"=w267) -> ()  [unwired: 2 in, 2 out]
              }
              frame #3 {
                # "Takes the decimal equivelant from the bit cluster and \nputs it into the \"Register\" array."
                n252 = local read "Reg_Numb"() -> (w277:i32)
                n253 = local read "Digital out"() -> (w279:u16)
                n254 = local read "Register"() -> (w278:u16[])
                n255 = Replace Array Subset(array=w278, new element=w279, index=w277) -> (w276:u16[])
                n256 = property on="Register" class="Arr (strict)"("Val(Sgnl)"=w276) -> ()  [unwired: 2 in, 2 out]
              }
              frame #4 {
                n257 = local read "Edited Register"() -> (w283:bool[])
                n258 = local read "Reg_Numb"() -> (w280:i32)
                n259 = Replace Array Subset(array=w283, new element=TRUE ("new element/subarray"), index=w280) -> (w281:bool[])
                n260 = property on="Edited Register" class="Arr (strict)"("Val(Sgnl)"=w281) -> ()  [unwired: 2 in, 2 out]
              }
            }
          }
          event "RAR trigger": Value Change; "Read All Reg": Mouse Up {
            n261 = event-data() -> ()  [unwired: 1 in, 4 out]
            n262 = stacked-sequence {
              frame #0 {
                n263 = property on="Status" class="Str"("Visible"=FALSE ("Front Panel Window:Resizeable")) -> ()  [unwired: 2 in, 2 out]
                n264 = property on="Progress" class="Slide (strict)"("Visible"=TRUE ("Front Panel Window:Resizeable")) -> ()  [unwired: 2 in, 2 out]
              }
              frame #1 {
                # "Call External \"Read All Reg\" VI"
                n265 = local read "USB DAQ Address"() -> (w290:i32)
                n266 = local read "Write I2C Address"() -> (w286:u8)
                n267 = local read "Register"() -> (w289:u16[])
                n268 = local read "Index to Reg No"() -> (w287:u8[])
                n269 = control-ref of="Progress"() -> (w291:refnum<vi>)
                n270 = call "Read_All_Reg.vi"("Register"=w289, "Slide Refnum"=w291, "USB DAQ Address"=w290, "Read I2C Address"=w286, "Index to Reg No"=w287) -> ("Output Register"=w292:u16[], "Status"=w288:string)
                n271 = property on="Register" class="Arr (strict)"("Val(Sgnl)"=w292) -> ()  [unwired: 2 in, 2 out]
                n272 = property on="Status" class="Str"("Val(Sgnl)"=w288) -> ()  [unwired: 2 in, 2 out]
              }
              frame #2 {
                # "Change status of registers to indicate that they have been written to"
                n273 = local read "Current History"() -> (w301:dbl[])
                n274 = local read "Shunt Voltage History"() -> (w303:dbl[])
                n275 = local read "Shunt Voltage"() -> (w304:dbl)
                n276 = local read "Current"() -> (w300:dbl)
                n277 = local read "Number of Registers"() -> (w308:i32)
                n278 = Insert Into Array(array=w303, new element=w304) -> (w302:dbl[])  [unwired: 1 in]
                n279 = Insert Into Array(array=w301, new element=w300) -> (w299:dbl[])  [unwired: 1 in]
                n280 = local write "Shunt Voltage History"(w302) -> ()
                n281 = local write "Current History"(w299) -> ()
                n282 = local write "Pending changes \nneed to be written"(FALSE ("Pending changes \nneed to be written")) -> ()
                n283 = Initialize Array(FALSE ("Boolean"), w308) -> (w306:bool[])
                n284 = local read "Bus Voltage History"() -> (w294:dbl[])
                n285 = local write "Edited Register"(w306) -> ()
                n286 = local read "Power History"() -> (w298:dbl[])
                n287 = local read "Bus Voltage"() -> (w295:dbl)
                n288 = local read "Power"() -> (w297:dbl)
                n289 = Insert Into Array(array=w294, new element=w295) -> (w293:dbl[])  [unwired: 1 in]
                n290 = Insert Into Array(array=w298, new element=w297) -> (w296:dbl[])  [unwired: 1 in]
                n291 = local write "Bus Voltage History"(w293) -> ()
                n292 = local write "Power History"(w296) -> ()
              }
              frame #3 {
                # "Remove all bold from table"
                n293 = local read "Number of Registers"() -> (w309:i32)
                n294 = for {
                  N: w309 -> [_]
                  i -> [w310]
                  n295 = for {
                    N: 4 -> [_]
                    tunnel: w310 -> [w312]
                    i -> [w313]
                    n296 = stacked-sequence {
                      tunnel: w313 -> [w317 _]
                      tunnel: w312 -> [w316 _]
                      frame #0 {
                        n297 = property on="Register Table" class="MCListbox (strict)"() -> ("ActiveCell"=w315:T13)  [unwired: 2 in, 2 out]
                        n298 = Bundle By Name(cluster=w315, "Row"=w316, "Column"=w317) -> (w314:T13)
                        n299 = property on="Register Table" class="MCListbox (strict)"("ActiveCell"=w314) -> ()  [unwired: 2 in, 2 out]
                      }
                      frame #1 {
                        n300 = property on="Register Table" class="MCListbox (strict)"("CellFontBold"=FALSE ("Active Cell:Cell Font:Bold")) -> ()  [unwired: 2 in, 2 out]
                      }
                    }
                  }
                }
              }
              frame #4 {
                # "Update the Calculate Tab"
                n301 = local read "Graph Config"() -> (w319:T6)
                n302 = case shown="\"Power (W)\"" w319 {
                  frame "Vbus (V)", Default {
                    n303 = local read "Bus Voltage History"() -> (w323:dbl[])
                    n304 = local write "Waveform Graph"(w323) -> ()
                  }
                  frame "Vshunt (V)" {
                    n305 = local read "Shunt Voltage History"() -> (w324:dbl[])
                    n306 = local write "Waveform Graph"(w324) -> ()
                  }
                  frame "Current (A)" {
                    n307 = local read "Current History"() -> (w325:dbl[])
                    n308 = local write "Waveform Graph"(w325) -> ()
                  }
                  frame "Power (W)" {
                    n309 = local read "Power History"() -> (w326:dbl[])
                    n310 = local write "Waveform Graph"(w326) -> ()
                  }
                }
                n311 = local read "Calculate"() -> (w321:bool)
                n312 = Exclusive Or(1:w321, 2:TRUE ("Calculate")) -> (0:w320:bool)
                n313 = property on="Calculate" class="Bool (strict)"("Val(Sgnl)"=w320) -> ()  [unwired: 2 in, 2 out]
              }
              frame #5 {
                n314 = local read "Selected Path"() -> (w327:path)
                n315 = Not Equal?(x=w327, y=path "") -> (x != y?=w328:bool)
                n316 = case shown="True" w328 {
                  tunnel: w327 -> [_ w337]
                  frame False {
                  }
                  frame True {
                    n317 = call "Elapsed Time"() -> ("Present (s)"=w339:dbl)  [unwired: 12 in, 7 out]
                    n318 = local read "Bus Voltage"() -> (w335:dbl)
                    n319 = local read "Shunt Voltage"() -> (w334:dbl)
                    n320 = local read "Current"() -> (w333:dbl)
                    n321 = local read "Power"() -> (w332:dbl)
                    n322 = local read "Initial Time"() -> (w338:dbl)
                    n323 = Subtract(x=w339, y=w338) -> (x-y=w336:dbl)
                    n324 = Build Array(w336, w335, w334, w333, w332) -> (w331:dbl[])
                    n325 = call-poly <vilib>:"Write To Spreadsheet File.vi"("delimiter (\\t)"="," ("delimiter (\\t)"), "format (%.3f)"="%#g", "append to file? (new file:F)"=TRUE, "1D data"=w331, "file path (dialog if empty)"=w337) -> ()  [unwired: 3 in, 1 out]
                  }
                }
              }
            }
          }
          event "Write All Reg": Mouse Up {
            n326 = event-data() -> ()  [unwired: 1 in, 8 out]
            n327 = stacked-sequence {
              frame #0 {
                n328 = local read "Operating Mode"() -> (w342:T4)
                n329 = property on="Status" class="Str"("Visible"=FALSE ("Front Panel Window:Resizeable")) -> ()  [unwired: 2 in, 2 out]
                n330 = property on="Progress" class="Slide (strict)"("Visible"=TRUE ("Front Panel Window:Resizeable")) -> ()  [unwired: 2 in, 2 out]
                n331 = case shown="\"Power Down \"" w342 {
                  frame "Power Down", Default {
                  }
                  frame "Shunt Voltage, Triggered" {
                    w347 = u16 0  # Reg Number
                    n332 = local read "Edited Register"() -> (w346:bool[])
                    n333 = Replace Array Subset(array=w346, new element=TRUE ("new element/subarray"), index=w347) -> (w345:bool[])
                    n334 = property on="Edited Register" class="Arr (strict)"("Val(Sgnl)"=w345) -> ()  [unwired: 2 in, 2 out]
                  }
                  frame "Bus Voltage, Triggered" {
                    w351 = u16 0  # Reg Number
                    n335 = local read "Edited Register"() -> (w350:bool[])
                    n336 = Replace Array Subset(array=w350, new element=TRUE ("new element/subarray"), index=w351) -> (w349:bool[])
                    n337 = property on="Edited Register" class="Arr (strict)"("Val(Sgnl)"=w349) -> ()  [unwired: 2 in, 2 out]
                  }
                  frame "Shunt and Bus, Triggered" {
                    w355 = u16 0  # Reg Number
                    n338 = local read "Edited Register"() -> (w354:bool[])
                    n339 = Replace Array Subset(array=w354, new element=TRUE ("new element/subarray"), index=w355) -> (w353:bool[])
                    n340 = property on="Edited Register" class="Arr (strict)"("Val(Sgnl)"=w353) -> ()  [unwired: 2 in, 2 out]
                  }
                  frame "Power Down " {
                  }
                  frame "Shunt Voltage, Continuous" {
                  }
                  frame "Bus Voltage, Continuous" {
                  }
                  frame "Shunt and Bus, Continuous" {
                  }
                }
              }
              frame #1 {
                # "Call external \"Write All Reg\" VI"
                n341 = local read "USB DAQ Address"() -> (w360:i32)
                n342 = local read "Edited Register"() -> (w363:bool[])
                n343 = control-ref of="Progress"() -> (w361:refnum<vi>)
                n344 = local read "Register"() -> (w362:u16[])
                n345 = local read "Index to Reg No"() -> (w357:u8[])
                n346 = call "Write_All_Reg.vi"("USB DAQ Address"=w360, "Write I2C Address"="Write I2C Address", "Edited Register"=w363, "Slide Refnum"=w361, "Index to Reg No"=w357, "Register"=w362) -> ("Status"=w358:string)
                n347 = property on="Status" class="Str"("Val(Sgnl)"=w358) -> ()  [unwired: 2 in, 2 out]
              }
              frame #2 {
                # "Change status of registers to indicate that they have been written to"
                n348 = local read "Number of Registers"() -> (w367:i32)
                n349 = local write "Pending changes \nneed to be written"(FALSE ("Pending changes \nneed to be written")) -> ()
                n350 = Initialize Array(FALSE ("Boolean"), w367) -> (w365:bool[])
                n351 = local write "Edited Register"(w365) -> ()
              }
              frame #3 {
                # "Remove all bold from table"
                n352 = local read "Number of Registers"() -> (w368:i32)
                n353 = for {
                  N: w368 -> [_]
                  i -> [w369]
                  n354 = for {
                    N: 4 -> [_]
                    tunnel: w369 -> [w371]
                    i -> [w372]
                    n355 = stacked-sequence {
                      tunnel: w372 -> [w376 _]
                      tunnel: w371 -> [w375 _]
                      frame #0 {
                        n356 = property on="Register Table" class="MCListbox (strict)"() -> ("ActiveCell"=w374:T13)  [unwired: 2 in, 2 out]
                        n357 = Bundle By Name(cluster=w374, "Row"=w375, "Column"=w376) -> (w373:T13)
                        n358 = property on="Register Table" class="MCListbox (strict)"("ActiveCell"=w373) -> ()  [unwired: 2 in, 2 out]
                      }
                      frame #1 {
                        n359 = property on="Register Table" class="MCListbox (strict)"("CellFontBold"=FALSE ("Active Cell:Cell Font:Bold")) -> ()  [unwired: 2 in, 2 out]
                      }
                    }
                  }
                }
              }
            }
          }
          event "Auto-Write": Value Change {
            n360 = event-data() -> ()  [unwired: 1 in, 6 out]
            n361 = local read "Auto-Write"() -> (w378:bool)
            n362 = case shown="True" w378 {
              frame False {
              }
              frame True {
                n363 = stacked-sequence {
                  frame #0 {
                    n364 = property on="Status" class="Str"("Visible"=FALSE ("Front Panel Window:Resizeable")) -> ()  [unwired: 2 in, 2 out]
                    n365 = property on="Progress" class="Slide (strict)"("Visible"=TRUE ("Front Panel Window:Resizeable")) -> ()  [unwired: 2 in, 2 out]
                  }
                  frame #1 {
                    # "Call external \"Write All Reg\" VI"
                    n366 = local read "Write I2C Address"() -> (w382:u8)
                    n367 = local read "USB DAQ Address"() -> (w384:i32)
                    n368 = local read "Edited Register"() -> (w387:bool[])
                    n369 = control-ref of="Progress"() -> (w385:refnum<vi>)
                    n370 = local read "Register"() -> (w386:u16[])
                    n371 = local read "Index to Reg No"() -> (w381:u8[])
                    n372 = call "Write_All_Reg.vi"("USB DAQ Address"=w384, "Write I2C Address"=w382, "Edited Register"=w387, "Slide Refnum"=w385, "Index to Reg No"=w381, "Register"=w386) -> ("Status"=w383:string)
                    n373 = property on="Status" class="Str"("Val(Sgnl)"=w383) -> ()  [unwired: 2 in, 2 out]
                  }
                  frame #2 {
                    # "Change status of registers to indicate that they have been written to"
                    n374 = local read "Number of Registers"() -> (w391:i32)
                    n375 = local write "Pending changes \nneed to be written"(FALSE ("Pending changes \nneed to be written")) -> ()
                    n376 = Initialize Array(FALSE ("Boolean"), w391) -> (w389:bool[])
                    n377 = local write "Edited Register"(w389) -> ()
                  }
                  frame #3 {
                    # "Remove all bold from table"
                    n378 = local read "Number of Registers"() -> (w392:i32)
                    n379 = for {
                      N: w392 -> [_]
                      i -> [w393]
                      n380 = for {
                        N: 4 -> [_]
                        tunnel: w393 -> [w395]
                        i -> [w396]
                        n381 = stacked-sequence {
                          tunnel: w396 -> [w400 _]
                          tunnel: w395 -> [w399 _]
                          frame #0 {
                            n382 = property on="Register Table" class="MCListbox (strict)"() -> ("ActiveCell"=w398:T13)  [unwired: 2 in, 2 out]
                            n383 = Bundle By Name(cluster=w398, "Row"=w399, "Column"=w400) -> (w397:T13)
                            n384 = property on="Register Table" class="MCListbox (strict)"("ActiveCell"=w397) -> ()  [unwired: 2 in, 2 out]
                          }
                          frame #1 {
                            n385 = property on="Register Table" class="MCListbox (strict)"("CellFontBold"=FALSE ("Active Cell:Cell Font:Bold")) -> ()  [unwired: 2 in, 2 out]
                          }
                        }
                      }
                    }
                  }
                }
              }
            }
          }
          event "A0": Value Change {
            # "A0 represents the 2nd and 3rd bit of the I2C Address\nSee Table 1 in the INA226 datatsheet for explanation"
            n386 = event-data() -> ()  [unwired: 1 in, 6 out]
            n387 = local read "Write I2C Address"() -> (w410:u8)
            n388 = Logical Shift(y=i8 1, x="A0") -> (x << y=w407:u8)
            n389 = And(x=u8 248 ("y"), y=w410) -> (x .and. y?=w408:u8)
            n390 = Or(x=w407, y=w408) -> (x .or. y?=w404:u8)
            n391 = local write "Write I2C Address"(w404) -> ()
            n392 = Logical Shift(y=i8 -1, x=w404) -> (x << y=w405:u8)
            n393 = local write "I2C Address"(w405) -> ()
          }
          event "A1": Value Change {
            # "A1 represents the 4th and 5th bit of the I2C Write Address\nSee Table 1 in the INA226 datatsheet for explanation"
            n394 = event-data() -> ()  [unwired: 1 in, 6 out]
            n395 = local read "Write I2C Address"() -> (w419:u8)
            n396 = Logical Shift(y=i8 3, x="A1") -> (x << y=w416:u8)
            n397 = And(x=u8 230 ("y"), y=w419) -> (x .and. y?=w417:u8)
            n398 = Or(x=w416, y=w417) -> (x .or. y?=w412:u8)
            n399 = local write "Write I2C Address"(w412) -> ()
            n400 = Logical Shift(y=i8 -1, x=w412) -> (x << y=→"I2C Address":u8)
          }
          event "Status": Value Change {
            n401 = event-data() -> ()  [unwired: 1 in, 6 out]
            n402 = local read "Status"() -> (w422:string)
            n403 = Equal?(x=w422, y="") -> (x = y?=w420:bool)
            n404 = case shown="True" w420 {
              frame False {
                n405 = property on="Status" class="Str"("Visible"=TRUE ("Front Panel Window:Resizeable")) -> ()  [unwired: 2 in, 2 out]
                n406 = property on="Progress" class="Slide (strict)"("Visible"=FALSE ("Front Panel Window:Resizeable")) -> ()  [unwired: 2 in, 2 out]
              }
              frame True {
                n407 = property on="Progress" class="Slide (strict)"("Visible"=TRUE ("Front Panel Window:Resizeable")) -> ()  [unwired: 2 in, 2 out]
                n408 = property on="Status" class="Str"("Visible"=FALSE ("Front Panel Window:Resizeable")) -> ()  [unwired: 2 in, 2 out]
              }
            }
          }
          event "Power": Mouse Up {
            n409 = event-data() -> ()  [unwired: 1 in, 8 out]
            n410 = case shown="True" "Power" {
              frame False {
                n411 = local read "PORT2"() -> (w429:i16)
                n412 = call "SM_VDUT ON-OFF.vi"("Port2 IN"=w429, "Power State"=enum16{"Vdut On", "Vdut Off"}."Vdut Off") -> ("Port2 OUT"=w428:u8)  [unwired: 1 in, 1 out]
                n413 = local write "PORT2"(w428) -> ()
              }
              frame True {
                w432 = 0.0 ("Enter Current LSB")
                n414 = local read "Enter Rshunt \nVariables"() -> (w433:cluster{"Max Current":dbl, "Resistance":dbl})
                n415 = local write "Enter Current LSB"(w432) -> ()
                n416 = local write "Low LSB"(w432) -> ()
                n417 = local write "High LSB"(w432) -> ()
                n418 = Bundle By Name(cluster=w433, "Max Current"=w432, "Resistance"=w432) -> (w434:cluster{"Max Current":dbl, "Resistance":dbl})
                n419 = local write "Enter Rshunt \nVariables"(w434) -> ()
                n420 = local read "PORT2"() -> (w436:i16)
                n421 = call "SM_VDUT ON-OFF.vi"("Port2 IN"=w436, "Power State"=enum16{"Vdut On", "Vdut Off"}."Vdut On") -> ("Port2 OUT"=w435:u8)  [unwired: 1 in, 1 out]
                n422 = local write "PORT2"(w435) -> ()
                n423 = property on="RAR trigger" class="Bool (strict)"("Val(Sgnl)"=TRUE) -> ()  [unwired: 2 in, 2 out]
              }
            }
          }
          event "Operating Mode": Value Change {
            n424 = event-data() -> ()  [unwired: 1 in, 6 out]
            n425 = flat-sequence {
              frame #0 {
                w440 = u16 3  # Word Length
                w441 = u16 0  # Bit Number
                w442 = u16 0  # Reg Number
                n426 = local read "Operating Mode"() -> (w438:T4)
                n427 = local read "Register"() -> (w443:u16[])
                n428 = call "Change_Bits_in_Reg.vi"("Reg Number"=w442, "Bit Number"=w441, "Word Length"=w440, "Bit Word In"=w438, "Reg In"=w443) -> ("Reg Out"=w439:u16[])
                n429 = property on="Register" class="Arr (strict)"("Val(Sgnl)"=w439) -> ()  [unwired: 2 in, 2 out]
              }
              frame #1 {
                w446 = u16 0  # Reg Number
                n430 = local read "Edited Register"() -> (w445:bool[])
                n431 = Replace Array Subset(array=w445, new element=TRUE ("new element/subarray"), index=w446) -> (w444:bool[])
                n432 = property on="Edited Register" class="Arr (strict)"("Val(Sgnl)"=w444) -> ()  [unwired: 2 in, 2 out]
              }
            }
          }
          event "Bus Voltage Conversion Time": Value Change {
            n433 = event-data() -> ()  [unwired: 1 in, 6 out]
            n434 = flat-sequence {
              frame #0 {
                w450 = u16 3  # Word Length
                w451 = u16 6  # Bit Number
                w452 = u16 0  # Reg Number
                n435 = local read "Bus Voltage Conversion Time"() -> (w448:T3)
                n436 = local read "Register"() -> (w453:u16[])
                n437 = call "Change_Bits_in_Reg.vi"("Reg Number"=w452, "Bit Number"=w451, "Word Length"=w450, "Bit Word In"=w448, "Reg In"=w453) -> ("Reg Out"=w449:u16[])
                n438 = property on="Register" class="Arr (strict)"("Val(Sgnl)"=w449) -> ()  [unwired: 2 in, 2 out]
              }
              frame #1 {
                w456 = u16 0  # Reg Number
                n439 = local read "Edited Register"() -> (w455:bool[])
                n440 = Replace Array Subset(array=w455, new element=TRUE ("new element/subarray"), index=w456) -> (w454:bool[])
                n441 = property on="Edited Register" class="Arr (strict)"("Val(Sgnl)"=w454) -> ()  [unwired: 2 in, 2 out]
              }
            }
          }
          event "Conversion Ready": Mouse Up {
            n442 = event-data() -> ()  [unwired: 1 in, 8 out]
            n443 = flat-sequence {
              frame #0 {
                w461 = u16 1  # Word Length
                w462 = u16 10  # Bit Number
                w463 = u16 6  # Reg Number
                n444 = local read "Conversion Ready"() -> (w459:bool)
                n445 = local read "Register"() -> (w464:u16[])
                n446 = Boolean To (0,1)(Boolean=w459) -> (0, 1=w458:i16)
                n447 = call "Change_Bits_in_Reg.vi"("Reg Number"=w463, "Bit Number"=w462, "Word Length"=w461, "Bit Word In"=w458, "Reg In"=w464) -> ("Reg Out"=w460:u16[])
                n448 = property on="Register" class="Arr (strict)"("Val(Sgnl)"=w460) -> ()  [unwired: 2 in, 2 out]
              }
              frame #1 {
                w467 = u16 6  # Reg Number
                n449 = local read "Edited Register"() -> (w466:bool[])
                n450 = Replace Array Subset(array=w466, new element=TRUE ("new element/subarray"), index=w467) -> (w465:bool[])
                n451 = property on="Edited Register" class="Arr (strict)"("Val(Sgnl)"=w465) -> ()  [unwired: 2 in, 2 out]
              }
            }
          }
          event "Alert Limit": Value Change {
            n452 = event-data() -> ()  [unwired: 1 in, 6 out]
            n453 = stacked-sequence {
              frame #0 {
                n454 = local read "Alert Config"() -> (w469:T2)
                n455 = case shown="\"None\"" w469 {
                  frame "Over-Limit Power", Default {
                    # "Divide the Limit by the Bus Voltage LSB:current LSB *25"
                    n456 = local read "Enter Current LSB"() -> (w477:dbl)
                    n457 = property on="Alert Limit" class="DigNum (strict)"("FormatString"="%#_4pW" ("Format String")) -> ()  [unwired: 2 in, 2 out]
                    n458 = local read "Alert Limit"() -> (w476:dbl)
                    n459 = Multiply(x=25.0, y=w477) -> (x*y=w472:dbl)
                    n460 = Divide(x=w476, y=w472) -> (x/y=w471:dbl)
                    n461 = Multiply(x=w472, y=2e+16) -> (x*y=w474:dbl)
                    n462 = To Unsigned Word Integer(number=w471) -> (unsigned 16bit integer=w470:u16)
                    n463 = local write "Alert Limit Digital"(w470) -> ()
                    n464 = property on="Alert Limit" class="DigNum (strict)"("Minimum"=0.0 ("Data Entry Limits:Minimum")) -> ()  [unwired: 2 in, 2 out]
                    n465 = property on="Alert Limit" class="DigNum (strict)"("Maximum"=w474) -> ()  [unwired: 2 in, 2 out]
                  }
                  frame "Bus Voltage Over-Voltage" {
                    w485 = 0.00125 ("y")
                    # "Divide the Limit by the Bus Voltage LSB: 1.25ma"
                    n466 = property on="Alert Limit" class="DigNum (strict)"("FormatString"="%#_4pV" ("Format String")) -> ()  [unwired: 2 in, 2 out]
                    n467 = local read "Alert Limit"() -> (w487:dbl)
                    n468 = Divide(x=w487, y=w485) -> (x/y=w481:dbl)
                    n469 = Multiply(x=w485, y=2000000000000000.0) -> (x*y=w482:dbl)
                    n470 = To Unsigned Word Integer(number=w481) -> (unsigned 16bit integer=w480:u16)
                    n471 = local write "Alert Limit Digital"(w480) -> ()
                    n472 = property on="Alert Limit" class="DigNum (strict)"("Minimum"=0.0 ("Data Entry Limits:Minimum")) -> ()  [unwired: 2 in, 2 out]
                    n473 = property on="Alert Limit" class="DigNum (strict)"("Maximum"=w482) -> ()  [unwired: 2 in, 2 out]
                  }
                  frame "Shunt Voltage Under-Voltage" {
                    w493 = 2.5e-06 ("y")
                    # "Divide the Limit by the Shunt Voltage LSB: 2.5uV"
                    n474 = property on="Alert Limit" class="DigNum (strict)"("FormatString"="%#_4pV" ("Format String")) -> ()  [unwired: 2 in, 2 out]
                    n475 = local read "Alert Limit"() -> (w496:dbl)
                    n476 = Divide(x=w496, y=w493) -> (x/y=w489:dbl)
                    n477 = Multiply(x=w493, y=2000000000000000.0) -> (x*y=w492:dbl)
                    n478 = To Word Integer(number=w489) -> (16bit integer=w488:i16)
                    n479 = local write "Alert Limit Digital"(w488) -> ()
                    n480 = Multiply(x=-1.0, y=w492) -> (x*y=w490:dbl)
                    n481 = property on="Alert Limit" class="DigNum (strict)"("Minimum"=w490) -> ()  [unwired: 2 in, 2 out]
                    n482 = property on="Alert Limit" class="DigNum (strict)"("Maximum"=w492) -> ()  [unwired: 2 in, 2 out]
                  }
                  frame "Shunt Voltage Over-Voltage" {
                    w499 = 2.5e-06 ("y")
                    # "Divide the Limit by the Shunt Voltage LSB: 2.5uV"
                    n483 = property on="Alert Limit" class="DigNum (strict)"("FormatString"="%#_4pV" ("Format String")) -> ()  [unwired: 2 in, 2 out]
                    n484 = local read "Alert Limit"() -> (w505:dbl)
                    n485 = Divide(x=w505, y=w499) -> (x/y=w498:dbl)
                    n486 = Multiply(x=w499, y=2000000000000000.0) -> (x*y=w502:dbl)
                    n487 = To Word Integer(number=w498) -> (16bit integer=w497:i16)
                    n488 = Multiply(x=-1.0, y=w502) -> (x*y=w500:dbl)
                    n489 = local write "Alert Limit Digital"(w497) -> ()
                    n490 = property on="Alert Limit" class="DigNum (strict)"("Minimum"=w500) -> ()  [unwired: 2 in, 2 out]
                    n491 = property on="Alert Limit" class="DigNum (strict)"("Maximum"=w502) -> ()  [unwired: 2 in, 2 out]
                  }
                  frame "Bus Voltage Under-Voltage" {
                    w509 = 0.00125 ("y")
                    # "Divide the Limit by the Bus Voltage LSB: 1.25ma"
                    n492 = property on="Alert Limit" class="DigNum (strict)"("FormatString"="%#_4pV" ("Format String")) -> ()  [unwired: 2 in, 2 out]
                    n493 = local read "Alert Limit"() -> (w513:dbl)
                    n494 = Multiply(x=w509, y=2000000000000000.0) -> (x*y=w510:dbl)
                    n495 = Divide(x=w513, y=w509) -> (x/y=w507:dbl)
                    n496 = To Unsigned Word Integer(number=w507) -> (unsigned 16bit integer=w506:u16)
                    n497 = local write "Alert Limit Digital"(w506) -> ()
                    n498 = property on="Alert Limit" class="DigNum (strict)"("Minimum"=0.0 ("Data Entry Limits:Minimum")) -> ()  [unwired: 2 in, 2 out]
                    n499 = property on="Alert Limit" class="DigNum (strict)"("Maximum"=w510) -> ()  [unwired: 2 in, 2 out]
                  }
                  frame "None" {
                    n500 = property on="Alert Limit" class="DigNum (strict)"("FormatString"="%#" ("Format String")) -> ()  [unwired: 2 in, 2 out]
                    n501 = local write "Alert Limit Digital"(i16 0 ("Alert Limit Digital")) -> ()
                    n502 = property on="Alert Limit" class="DigNum (strict)"("Minimum"=0.0 ("Data Entry Limits:Minimum")) -> ()  [unwired: 2 in, 2 out]
                    n503 = property on="Alert Limit" class="DigNum (strict)"("Maximum"=0.0 ("Data Entry Limits:Maximum")) -> ()  [unwired: 2 in, 2 out]
                  }
                }
              }
              frame #1 {
                n504 = flat-sequence {
                  frame #0 {
                    w520 = u16 16  # Word Length
                    w521 = u16 0  # Bit Number
                    w522 = u16 7  # Reg Number
                    n505 = local read "Alert Limit Digital"() -> (w518:i16)
                    n506 = local read "Register"() -> (w523:u16[])
                    n507 = call "Change_Bits_in_Reg.vi"("Reg Number"=w522, "Bit Number"=w521, "Word Length"=w520, "Bit Word In"=w518, "Reg In"=w523) -> ("Reg Out"=w519:u16[])
                    n508 = property on="Register" class="Arr (strict)"("Val(Sgnl)"=w519) -> ()  [unwired: 2 in, 2 out]
                  }
                  frame #1 {
                    w526 = u16 7  # Reg Number
                    n509 = local read "Edited Register"() -> (w525:bool[])
                    n510 = Replace Array Subset(array=w525, new element=TRUE ("new element/subarray"), index=w526) -> (w524:bool[])
                    n511 = property on="Edited Register" class="Arr (strict)"("Val(Sgnl)"=w524) -> ()  [unwired: 2 in, 2 out]
                  }
                }
              }
            }
          }
          event "Alert Config": Value Change {
            n512 = event-data() -> ()  [unwired: 1 in, 6 out]
            n513 = flat-sequence {
              frame #0 {
                # "Change the Digital Alert Limit\nThis changes based on the \nAlert Config bits"
                n514 = local read "Alert Limit"() -> (w528:dbl)
                n515 = property on="Alert Limit" class="DigNum (strict)"("Val(Sgnl)"=w528) -> ()  [unwired: 2 in, 2 out]
              }
              frame #1 {
                w533 = u16 5  # Word Length
                w534 = u16 11  # Bit Number
                w535 = u16 6  # Reg Number
                # "These bits can only be triggered one at a time"
                n516 = local read "Register"() -> (w536:u16[])
                n517 = Logical Shift(y="Alert Config", x=u32 1) -> (x << y=w530:u32)
                n518 = call "Change_Bits_in_Reg.vi"("Reg Number"=w535, "Bit Number"=w534, "Word Length"=w533, "Bit Word In"=w530, "Reg In"=w536) -> ("Reg Out"=w532:u16[])
                n519 = property on="Register" class="Arr (strict)"("Val(Sgnl)"=w532) -> ()  [unwired: 2 in, 2 out]
              }
              frame #2 {
                w539 = u16 6  # Reg Number
                n520 = local read "Edited Register"() -> (w538:bool[])
                n521 = Replace Array Subset(array=w538, new element=TRUE ("new element/subarray"), index=w539) -> (w537:bool[])
                n522 = property on="Edited Register" class="Arr (strict)"("Val(Sgnl)"=w537) -> ()  [unwired: 2 in, 2 out]
              }
            }
          }
          event "Averaging Mode": Value Change {
            n523 = event-data() -> ()  [unwired: 1 in, 6 out]
            n524 = flat-sequence {
              frame #0 {
                w543 = u16 3  # Word Length
                w544 = u16 9  # Bit Number
                w545 = u16 0  # Reg Number
                n525 = local read "Averaging Mode"() -> (w541:T5)
                n526 = local read "Register"() -> (w546:u16[])
                n527 = call "Change_Bits_in_Reg.vi"("Reg Number"=w545, "Bit Number"=w544, "Word Length"=w543, "Bit Word In"=w541, "Reg In"=w546) -> ("Reg Out"=w542:u16[])
                n528 = property on="Register" class="Arr (strict)"("Val(Sgnl)"=w542) -> ()  [unwired: 2 in, 2 out]
              }
              frame #1 {
                w549 = u16 0  # Reg Number
                n529 = local read "Edited Register"() -> (w548:bool[])
                n530 = Replace Array Subset(array=w548, new element=TRUE ("new element/subarray"), index=w549) -> (w547:bool[])
                n531 = property on="Edited Register" class="Arr (strict)"("Val(Sgnl)"=w547) -> ()  [unwired: 2 in, 2 out]
              }
            }
          }
          event "Shunt Voltage Conversion Time": Value Change {
            n532 = event-data() -> ()  [unwired: 1 in, 6 out]
            n533 = flat-sequence {
              frame #0 {
                w553 = u16 3  # Word Length
                w554 = u16 3  # Bit Number
                w555 = u16 0  # Reg Number
                n534 = local read "Shunt Voltage Conversion Time"() -> (w551:T3)
                n535 = local read "Register"() -> (w556:u16[])
                n536 = call "Change_Bits_in_Reg.vi"("Reg Number"=w555, "Bit Number"=w554, "Word Length"=w553, "Bit Word In"=w551, "Reg In"=w556) -> ("Reg Out"=w552:u16[])
                n537 = property on="Register" class="Arr (strict)"("Val(Sgnl)"=w552) -> ()  [unwired: 2 in, 2 out]
              }
              frame #1 {
                w559 = u16 0  # Reg Number
                n538 = local read "Edited Register"() -> (w558:bool[])
                n539 = Replace Array Subset(array=w558, new element=TRUE ("new element/subarray"), index=w559) -> (w557:bool[])
                n540 = property on="Edited Register" class="Arr (strict)"("Val(Sgnl)"=w557) -> ()  [unwired: 2 in, 2 out]
              }
            }
          }
          event "Register Table": Value Change {
            n541 = event-data() -> ("NewVal"=w561:i32)  [unwired: 1 in, 5 out]
            n542 = stacked-sequence {
              tunnel: w561 -> [w566 w579 w595]
              frame #0 {
                # "This frame changes the labels above each cluster -bit when \nthe row in the register changes"
                n543 = local read "bit_text_array"() -> (w567:string[][])
                n544 = local read "Numb_Bits_In_Reg"() -> (w564:i32)
                n545 = Index Array(array=w567, index (row)=w566) -> (element=w568:string[])  [unwired: 1 in]
                n546 = Equal?(x=w564, y=16) -> (x = y?=w562:bool)
                n547 = case shown="False" w562 {
                  tunnel: [w569 w570] -> w565
                  frame False {
                    n548 = property on="dig_bits8" class="Clust (strict)"() -> ("Controls[]"=w569:refnum<vi>[])  [unwired: 2 in, 2 out]
                  }
                  frame True {
                    n549 = property on="dig_bits 16" class="Clust (strict)"() -> ("Controls[]"=w570:refnum<vi>[])  [unwired: 2 in, 2 out]
                  }
                }
                n550 = for {
                  tunnel: w568 -> [w572] mode=indexing
                  tunnel: w565 -> [w571] mode=indexing
                  n551 = property class="Ctl"(reference=w571, "Caption.Text"=w572) -> ()  [unwired: 1 in, 2 out]
                }
                "Reg_Numb" <- w566
              }
              frame #1 {
                # "This frame updates the bits in the cluster acording the the \n\"Register\" array."
                n552 = local read "Register"() -> (w578:u16[])
                n553 = local read "Numb_Bits_In_Reg"() -> (w577:i32)
                n554 = Index Array(array=w578, index=w579) -> (element=w580:u16)
                n555 = for {
                  N: w577 -> [_]
                  tunnel: [w586] -> w573 mode=indexing
                  shift-right: [w585] -> _
                  shift-left: w580 -> [w587]
                  n556 = Quotient & Remainder(x=w587, y=u8 2) -> (x-y*floor(x/y)=w586:u16, floor(x/y)=w585:u16)
                }
                n557 = local read "Numb_Bits_In_Reg"() -> (w576:i32)
                n558 = Equal?(x=w576, y=16) -> (x = y?=w574:bool)
                n559 = case shown="True" w574 {
                  tunnel: w573 -> [w582 w584]
                  frame False {
                    n560 = Array To Cluster(array=w582) -> (cluster=w581:T14)
                    n561 = property on="dig_bits8" class="Clust (strict)"("Value"=w581) -> ()  [unwired: 2 in, 2 out]
                  }
                  frame True {
                    n562 = Array To Cluster(array=w584) -> (cluster=w583:T15)
                    n563 = property on="dig_bits 16" class="Clust (strict)"("Value"=w583) -> ()  [unwired: 2 in, 2 out]
                  }
                }
              }
              frame #2 {
                n564 = property on="Register Table" class="MCListbox (strict)"() -> ("ItemNames"=w593:string[][])  [unwired: 2 in, 2 out]
                n565 = Index Array(array=w593, index (row)=w595, index (col)=2 ("disabled index (col)")) -> (element=w590:string)
                n566 = call <vilib>:"Trim Whitespace.vi"("string"=w590) -> ("trimmed string"=w589:string)  [unwired: 1 in]
                n567 = Equal?(x="R", y=w589) -> (x = y?=w592:bool)
                n568 = case shown="True" w592 {
                  tunnel: w589 -> [w597 _]
                  frame False {
                    n569 = Equal?(x="R/W", y=w597) -> (x = y?=w596:bool)
                    n570 = case shown="True" w596 {
                      frame False {
                        n571 = One Button Dialog(message="Syntax error in table R/W.") -> ()  [unwired: 1 in, 1 out]
                      }
                      frame True {
                        w600 = u8 0 ("Disabled")
                        n572 = property on="dig_bits 16" class="Clust (strict)"("Disabled"=w600) -> ()  [unwired: 2 in, 2 out]
                        n573 = property on="dig_bits8" class="Clust (strict)"("Disabled"=w600) -> ()  [unwired: 2 in, 2 out]
                      }
                    }
                  }
                  frame True {
                    w601 = u8 1 ("Disabled")
                    n574 = property on="dig_bits 16" class="Clust (strict)"("Disabled"=w601) -> ()  [unwired: 2 in, 2 out]
                    n575 = property on="dig_bits8" class="Clust (strict)"("Disabled"=w601) -> ()  [unwired: 2 in, 2 out]
                  }
                }
              }
            }
          }
          event "Help w Reg": Mouse Up {
            n576 = event-data() -> ()  [unwired: 1 in, 8 out]
            n577 = local read "Reg_Numb"() -> (w602:i32)
            n578 = Current VI's Path() -> (path=w603:path)
            n579 = call "Help_w_Reg.vi"("Reg No"=w602, "App Path"=w603) -> ()  [unwired: 1 in]
          }
          event "Edited Register": Value Change {
            n580 = event-data() -> ("NewVal"=w605:bool[])  [unwired: 1 in, 5 out]
            n581 = local read "Auto-Write"() -> (w604:bool)
            n582 = case shown="False" w604 {
              tunnel: w605 -> [w606 _]
              frame False {
                n583 = for {
                  tunnel: w606 -> [w607] mode=indexing
                  i -> [w608]
                  n584 = case shown="True" w607 {
                    tunnel: w608 -> [_ w610]
                    frame False {
                    }
                    frame True {
                      n585 = for {
                        N: 4 -> [_]
                        tunnel: w610 -> [w612]
                        i -> [w613]
                        n586 = stacked-sequence {
                          tunnel: w613 -> [w617 _]
                          tunnel: w612 -> [w616 _]
                          frame #0 {
                            n587 = property on="Register Table" class="MCListbox (strict)"() -> ("ActiveCell"=w615:T13)  [unwired: 2 in, 2 out]
                            n588 = Bundle By Name(cluster=w615, "Row"=w616, "Column"=w617) -> (w614:T13)
                            n589 = property on="Register Table" class="MCListbox (strict)"("ActiveCell"=w614) -> ()  [unwired: 2 in, 2 out]
                          }
                          frame #1 {
                            n590 = property on="Register Table" class="MCListbox (strict)"("CellFontBold"=TRUE ("Active Cell:Cell Font:Bold")) -> ()  [unwired: 2 in, 2 out]
                          }
                        }
                      }
                      "Pending changes \nneed to be written" <- TRUE ("Pending changes \nneed to be written")
                    }
                  }
                }
              }
              frame True {
              }
            }
          }
          event "Register": Value Change {
            n591 = event-data() -> ()  [unwired: 1 in, 6 out]
            n592 = stacked-sequence {
              frame #0 {
                n593 = stacked-sequence {
                  frame #0 {
                    w620 = u16 3  # Word Length
                    w621 = u16 0  # Bit Number
                    w622 = u16 0  # Reg Number
                    n594 = local read "Register"() -> (w623:u16[])
                    n595 = call "Get_Bits_from_Reg.vi"("Word Length"=w620, "Bit Number"=w621, "Reg Number"=w622, "Reg_in"=w623) -> ("Bit Out"=w619:u16)
                    n596 = local write "Operating Mode"(w619) -> ()
                  }
                  frame #1 {
                    w625 = u16 3  # Word Length
                    w626 = u16 3  # Bit Number
                    w627 = u16 0  # Reg Number
                    n597 = local read "Register"() -> (w628:u16[])
                    n598 = call "Get_Bits_from_Reg.vi"("Word Length"=w625, "Bit Number"=w626, "Reg Number"=w627, "Reg_in"=w628) -> ("Bit Out"=w624:u16)
                    n599 = local write "Shunt Voltage Conversion Time"(w624) -> ()
                  }
                  frame #2 {
                    w630 = u16 3  # Word Length
                    w631 = u16 6  # Bit Number
                    w632 = u16 0  # Reg Number
                    n600 = local read "Register"() -> (w633:u16[])
                    n601 = call "Get_Bits_from_Reg.vi"("Word Length"=w630, "Bit Number"=w631, "Reg Number"=w632, "Reg_in"=w633) -> ("Bit Out"=w629:u16)
                    n602 = local write "Bus Voltage Conversion Time"(w629) -> ()
                  }
                  frame #3 {
                    w635 = u16 3  # Word Length
                    w636 = u16 9  # Bit Number
                    w637 = u16 0  # Reg Number
                    n603 = local read "Register"() -> (w638:u16[])
                    n604 = call "Get_Bits_from_Reg.vi"("Word Length"=w635, "Bit Number"=w636, "Reg Number"=w637, "Reg_in"=w638) -> ("Bit Out"=w634:u16)
                    n605 = local write "Averaging Mode"(w634) -> ()
                  }
                  frame #4 {
                    w648 = u16 16  # Word Length
                    w649 = u16 0  # Bit Number
                    w650 = u16 1  # Reg Number
                    n606 = local read "Register"() -> (w651:u16[])
                    n607 = call "Get_Bits_from_Reg.vi"("Word Length"=w648, "Bit Number"=w649, "Reg Number"=w650, "Reg_in"=w651) -> ("Bit Out"=w640:u16)
                    n608 = To Word Integer(number=w640) -> (16bit integer=w639:i16)
                    n609 = Multiply(x=w639, y=2.5e-06) -> (x*y=w643:dbl)
                    "Shunt Voltage" <- w643
                    n610 = Number To Decimal String(number=w643) -> (decimal integer string=w642:string)  [unwired: 1 in]
                    n611 = property on="Register Table" class="MCListbox (strict)"() -> ("ItemNames"=w645:string[][])  [unwired: 2 in, 2 out]
                    n612 = Replace Array Subset(array=w645, new element=w642, index (row)=1 ("disabled index (row)"), index (col)=3 ("disabled index (col)")) -> (w644:string[][])
                    n613 = property on="Register Table" class="MCListbox (strict)"("ItemNames"=w644) -> ()  [unwired: 2 in, 2 out]
                  }
                  frame #5 {
                    w655 = u16 16  # Word Length
                    w656 = u16 0  # Bit Number
                    w657 = u16 2  # Reg Number
                    n614 = local read "Register"() -> (w658:u16[])
                    n615 = call "Get_Bits_from_Reg.vi"("Word Length"=w655, "Bit Number"=w656, "Reg Number"=w657, "Reg_in"=w658) -> ("Bit Out"=w652:u16)
                    n616 = Multiply(x=w652, y=0.00125) -> (x*y=→"Bus Voltage":dbl)
                  }
                  frame #6 {
                    w663 = u16 16  # Word Length
                    w664 = u16 0  # Bit Number
                    w665 = u16 4  # Reg Number
                    # "Calculate the LSB by using eqn in datasheet:\nVshunt*Calibration/2048 = Current"
                    n617 = local read "Register"() -> (w666:u16[])
                    n618 = call "Get_Bits_from_Reg.vi"("Word Length"=w663, "Bit Number"=w664, "Reg Number"=w665, "Reg_in"=w666) -> ("Bit Out"=w660:u16)
                    n619 = local read "Enter Current LSB"() -> (w661:dbl)
                    n620 = To Word Integer(number=w660) -> (16bit integer=w659:i16)
                    n621 = Multiply(x=w659, y=w661) -> (x*y=→"Current":dbl)
                  }
                  frame #7 {
                    w672 = u16 16  # Word Length
                    w673 = u16 0  # Bit Number
                    w674 = u16 3  # Reg Number
                    # "Calculate the LSB by using eqn in datasheet:\n25*1x10-3 Current LSB = Power"
                    n622 = local read "Register"() -> (w675:u16[])
                    n623 = call "Get_Bits_from_Reg.vi"("Word Length"=w672, "Bit Number"=w673, "Reg Number"=w674, "Reg_in"=w675) -> ("Bit Out"=w669:u16)
                    n624 = local read "Enter Current LSB"() -> (w670:dbl)
                    n625 = Multiply(x=25.0, y=w670) -> (x*y=w667:dbl)
                    n626 = Multiply(x=w669, y=w667) -> (x*y=→"Power":dbl)
                  }
                  frame #8 {
                    w677 = u16 16  # Word Length
                    w678 = u16 0  # Bit Number
                    w679 = u16 5  # Reg Number
                    n627 = local read "Register"() -> (w680:u16[])
                    n628 = call "Get_Bits_from_Reg.vi"("Word Length"=w677, "Bit Number"=w678, "Reg Number"=w679, "Reg_in"=w680) -> ("Bit Out"=w676:u16)
                    n629 = local write "Enter Value for \nCalibration Register"(w676) -> ()
                  }
                  frame #9 {
                    w683 = u16 1  # Word Length
                    w684 = u16 3  # Bit Number
                    w685 = u16 6  # Reg Number
                    n630 = local read "Register"() -> (w686:u16[])
                    n631 = call "Get_Bits_from_Reg.vi"("Word Length"=w683, "Bit Number"=w684, "Reg Number"=w685, "Reg_in"=w686) -> ("Bit Out"=w682:u16)
                    n632 = call "Bit_to_Boolean.vi"("Bit In"=w682) -> ("Boolean Out"=→"Conv Ready Flag":bool)
                  }
                  frame #10 {
                    w689 = u16 1  # Word Length
                    w690 = u16 4  # Bit Number
                    w691 = u16 6  # Reg Number
                    n633 = local read "Register"() -> (w692:u16[])
                    n634 = call "Get_Bits_from_Reg.vi"("Word Length"=w689, "Bit Number"=w690, "Reg Number"=w691, "Reg_in"=w692) -> ("Bit Out"=w688:u16)
                    n635 = call "Bit_to_Boolean.vi"("Bit In"=w688) -> ("Boolean Out"=→"Alert":bool)
                  }
                  frame #11 {
                    w695 = u16 1  # Word Length
                    w696 = u16 10  # Bit Number
                    w697 = u16 6  # Reg Number
                    n636 = local read "Register"() -> (w698:u16[])
                    n637 = call "Get_Bits_from_Reg.vi"("Word Length"=w695, "Bit Number"=w696, "Reg Number"=w697, "Reg_in"=w698) -> ("Bit Out"=w694:u16)
                    n638 = call "Bit_to_Boolean.vi"("Bit In"=w694) -> ("Boolean Out"=w693:bool)
                    n639 = local write "Conversion Ready"(w693) -> ()
                  }
                  frame #12 {
                    w701 = u16 1  # Word Length
                    w702 = u16 11  # Bit Number
                    w703 = u16 6  # Reg Number
                    n640 = local read "Register"() -> (w704:u16[])
                    n641 = call "Get_Bits_from_Reg.vi"("Word Length"=w701, "Bit Number"=w702, "Reg Number"=w703, "Reg_in"=w704) -> ("Bit Out"=w700:u16)
                    n642 = call "Bit_to_Boolean.vi"("Bit In"=w700) -> ("Boolean Out"=w699:bool)
                    n643 = case shown="False" w699 {
                      frame False {
                        n644 = local write "Alert Config"(T2."None" ("Alert Config")) -> ()
                      }
                      frame True {
                        n645 = property on="Alert Limit" class="DigNum (strict)"("FormatString"="%#_4pW" ("Format String")) -> ()  [unwired: 2 in, 2 out]
                        n646 = local write "Alert Config"(T11."Over-Limit Power" ("Alert Config")) -> ()
                      }
                    }
                  }
                  frame #13 {
                    w710 = u16 1  # Word Length
                    w711 = u16 12  # Bit Number
                    w712 = u16 6  # Reg Number
                    n647 = local read "Register"() -> (w713:u16[])
                    n648 = call "Get_Bits_from_Reg.vi"("Word Length"=w710, "Bit Number"=w711, "Reg Number"=w712, "Reg_in"=w713) -> ("Bit Out"=w709:u16)
                    n649 = call "Bit_to_Boolean.vi"("Bit In"=w709) -> ("Boolean Out"=w708:bool)
                    n650 = case shown="True" w708 {
                      frame False {
                      }
                      frame True {
                        n651 = local write "Alert Config"(T11."Bus Voltage Under-Voltage" ("Alert Config")) -> ()
                      }
                    }
                  }
                  frame #14 {
                    w717 = u16 1  # Word Length
                    w718 = u16 13  # Bit Number
                    w719 = u16 6  # Reg Number
                    n652 = local read "Register"() -> (w720:u16[])
                    n653 = call "Get_Bits_from_Reg.vi"("Word Length"=w717, "Bit Number"=w718, "Reg Number"=w719, "Reg_in"=w720) -> ("Bit Out"=w716:u16)
                    n654 = call "Bit_to_Boolean.vi"("Bit In"=w716) -> ("Boolean Out"=w715:bool)
                    n655 = case shown="True" w715 {
                      frame False {
                      }
                      frame True {
                        n656 = local write "Alert Config"(T11."Bus Voltage Over-Voltage" ("Alert Config")) -> ()
                      }
                    }
                  }
                  frame #15 {
                    w724 = u16 1  # Word Length
                    w725 = u16 14  # Bit Number
                    w726 = u16 6  # Reg Number
                    n657 = local read "Register"() -> (w727:u16[])
                    n658 = call "Get_Bits_from_Reg.vi"("Word Length"=w724, "Bit Number"=w725, "Reg Number"=w726, "Reg_in"=w727) -> ("Bit Out"=w723:u16)
                    n659 = call "Bit_to_Boolean.vi"("Bit In"=w723) -> ("Boolean Out"=w722:bool)
                    n660 = case shown="True" w722 {
                      frame False {
                      }
                      frame True {
                        n661 = local write "Alert Config"(T11."Shunt Voltage Under-Voltage" ("Alert Config")) -> ()
                      }
                    }
                  }
                  frame #16 {
                    w731 = u16 1  # Word Length
                    w732 = u16 15  # Bit Number
                    w733 = u16 6  # Reg Number
                    n662 = local read "Register"() -> (w734:u16[])
                    n663 = call "Get_Bits_from_Reg.vi"("Word Length"=w731, "Bit Number"=w732, "Reg Number"=w733, "Reg_in"=w734) -> ("Bit Out"=w730:u16)
                    n664 = call "Bit_to_Boolean.vi"("Bit In"=w730) -> ("Boolean Out"=w729:bool)
                    n665 = case shown="True" w729 {
                      frame False {
                      }
                      frame True {
                        n666 = local write "Alert Config"(T11."Shunt Voltage Over-Voltage" ("Alert Config")) -> ()
                      }
                    }
                  }
                  frame #17 {
                    w737 = u16 16  # Word Length
                    w738 = u16 0  # Bit Number
                    w739 = u16 7  # Reg Number
                    n667 = local read "Register"() -> (w740:u16[])
                    n668 = call "Get_Bits_from_Reg.vi"("Word Length"=w737, "Bit Number"=w738, "Reg Number"=w739, "Reg_in"=w740) -> ("Bit Out"=w736:u16)
                    n669 = local write "Alert Limit Digital"(w736) -> ()
                  }
                }
              }
              frame #1 {
                n670 = local read "Alert Config"() -> (w741:T2)
                n671 = case shown="\"Over-Limit Power\", Default" w741 {
                  frame "Over-Limit Power", Default {
                    # "Divide the Limit by the Bus Voltage LSB:current LSB *25"
                    n672 = local read "Alert Limit Digital"() -> (w743:i16)
                    n673 = local read "Enter Current LSB"() -> (w750:dbl)
                    n674 = property on="Alert Limit" class="DigNum (strict)"("FormatString"="%#_4pW" ("Format String")) -> ()  [unwired: 2 in, 2 out]
                    n675 = To Unsigned Word Integer(number=w743) -> (unsigned 16bit integer=w742:u16)
                    n676 = Multiply(x=25.0, y=w750) -> (x*y=w746:dbl)
                    n677 = Multiply(x=w742, y=w746) -> (x*y=w745:dbl)
                    n678 = local write "Alert Limit"(w745) -> ()
                    n679 = Multiply(x=w746, y=2e+16) -> (x*y=w748:dbl)
                    n680 = property on="Alert Limit" class="DigNum (strict)"("Minimum"=0.0 ("Data Entry Limits:Minimum")) -> ()  [unwired: 2 in, 2 out]
                    n681 = property on="Alert Limit" class="DigNum (strict)"("Maximum"=w748) -> ()  [unwired: 2 in, 2 out]
                  }
                  frame "Bus Voltage Over-Voltage" {
                    w752 = 0.00125 ("y")
                    # "Divide the Limit by the Bus Voltage LSB: 1.25ma"
                    n682 = property on="Alert Limit" class="DigNum (strict)"("FormatString"="%#_4pV" ("Format String")) -> ()  [unwired: 2 in, 2 out]
                    n683 = local read "Alert Limit Digital"() -> (w754:i16)
                    n684 = Multiply(x=w752, y=2000000000000000.0) -> (x*y=w755:dbl)
                    n685 = Multiply(x=w754, y=w752) -> (x*y=w753:dbl)
                    n686 = local write "Alert Limit"(w753) -> ()
                    n687 = property on="Alert Limit" class="DigNum (strict)"("Minimum"=0.0 ("Data Entry Limits:Minimum")) -> ()  [unwired: 2 in, 2 out]
                    n688 = property on="Alert Limit" class="DigNum (strict)"("Maximum"=w755) -> ()  [unwired: 2 in, 2 out]
                  }
                  frame "Shunt Voltage Under-Voltage" {
                    w759 = 2.5e-06 ("y")
                    # "Divide the Limit by the Shunt Voltage LSB: 2.5uV"
                    n689 = property on="Alert Limit" class="DigNum (strict)"("FormatString"="%#_4pV" ("Format String")) -> ()  [unwired: 2 in, 2 out]
                    n690 = local read "Alert Limit Digital"() -> (w761:i16)
                    n691 = Multiply(x=w761, y=w759) -> (x*y=w760:dbl)
                    n692 = Multiply(x=w759, y=2000000000000000.0) -> (x*y=w764:dbl)
                    n693 = local write "Alert Limit"(w760) -> ()
                    n694 = Multiply(x=-1.0, y=w764) -> (x*y=w762:dbl)
                    n695 = property on="Alert Limit" class="DigNum (strict)"("Minimum"=w762) -> ()  [unwired: 2 in, 2 out]
                    n696 = property on="Alert Limit" class="DigNum (strict)"("Maximum"=w764) -> ()  [unwired: 2 in, 2 out]
                  }
                  frame "Shunt Voltage Over-Voltage" {
                    w767 = 2.5e-06 ("y")
                    # "Divide the Limit by the Shunt Voltage LSB: 2.5uV"
                    n697 = property on="Alert Limit" class="DigNum (strict)"("FormatString"="%#_4pV" ("Format String")) -> ()  [unwired: 2 in, 2 out]
                    n698 = local read "Alert Limit Digital"() -> (w769:i16)
                    n699 = Multiply(x=w767, y=2000000000000000.0) -> (x*y=w772:dbl)
                    n700 = Multiply(x=w769, y=w767) -> (x*y=w768:dbl)
                    n701 = Multiply(x=-1.0, y=w772) -> (x*y=w770:dbl)
                    n702 = local write "Alert Limit"(w768) -> ()
                    n703 = property on="Alert Limit" class="DigNum (strict)"("Minimum"=w770) -> ()  [unwired: 2 in, 2 out]
                    n704 = property on="Alert Limit" class="DigNum (strict)"("Maximum"=w772) -> ()  [unwired: 2 in, 2 out]
                  }
                  frame "Bus Voltage Under-Voltage" {
                    w775 = 0.00125 ("y")
                    # "Divide the Limit by the Bus Voltage LSB: 1.25ma"
                    n705 = property on="Alert Limit" class="DigNum (strict)"("FormatString"="%#_4pV" ("Format String")) -> ()  [unwired: 2 in, 2 out]
                    n706 = local read "Alert Limit Digital"() -> (w777:i16)
                    n707 = Multiply(x=w775, y=2000000000000000.0) -> (x*y=w779:dbl)
                    n708 = Multiply(x=w777, y=w775) -> (x*y=w776:dbl)
                    n709 = local write "Alert Limit"(w776) -> ()
                    n710 = property on="Alert Limit" class="DigNum (strict)"("Minimum"=0.0 ("Data Entry Limits:Minimum")) -> ()  [unwired: 2 in, 2 out]
                    n711 = property on="Alert Limit" class="DigNum (strict)"("Maximum"=w779) -> ()  [unwired: 2 in, 2 out]
                  }
                }
              }
              frame #2 {
                n712 = local read "Register"() -> (w782:u16[])
                n713 = for {
                  tunnel: w782 -> [w792] mode=indexing
                  i -> [w791]
                  # "This section is part of the shell.  It should not change in each project.\nThis updates the hex column of the table with the register values."
                  n714 = local read "Numb_Bits_In_Reg"() -> (w788:i32)
                  n715 = Number To Hexadecimal String(1:i16 4 ("width (-)"), 2:w792) -> (0:w785:string)
                  n716 = Equal?(x=w788, y=8) -> (x = y?=w786:bool)
                  n717 = case shown="True" w786 {
                    tunnel: w785 -> [w794 w797]
                    tunnel: [w794 w796] -> w784
                    frame False {
                    }
                    frame True {
                      n718 = String Subset(string=w797, offset (0)=2, length (rest)=2 ("length (rest)")) -> (substring=w796:string)
                    }
                  }
                  n719 = property on="Register Table" class="MCListbox (strict)"() -> ("ItemNames"=w790:string[][])  [unwired: 2 in, 2 out]
                  n720 = Replace Array Subset(array=w790, new element=w784, index (row)=w791, index (col)=3 ("disabled index (col)")) -> (w789:string[][])
                  n721 = property on="Register Table" class="MCListbox (strict)"("ItemNames"=w789) -> ()  [unwired: 2 in, 2 out]
                }
              }
              frame #3 {
                # "Reg_Numb is the current \nregister selected in the table"
                # "This section is part of the shell.  It should not change in each project.\nThis updates the bits in the bit cluster according to the current register selected in the table."
                n722 = local read "Reg_Numb"() -> (w804:i32)
                n723 = local read "Register"() -> (w805:u16[])
                n724 = local read "Numb_Bits_In_Reg"() -> (w799:i32)
                n725 = Index Array(array=w805, index=w804) -> (element=w806:u16)
                n726 = for {
                  N: w799 -> [_]
                  tunnel: [w812] -> w800 mode=indexing
                  shift-right: [w811] -> _
                  shift-left: w806 -> [w813]
                  n727 = Quotient & Remainder(x=w813, y=u8 2) -> (x-y*floor(x/y)=w812:u16, floor(x/y)=w811:u16)
                }
                n728 = local read "Numb_Bits_In_Reg"() -> (w803:i32)
                n729 = Equal?(x=w803, y=16) -> (x = y?=w801:bool)
                n730 = case shown="True" w801 {
                  tunnel: w800 -> [w808 w810]
                  frame False {
                    n731 = Array To Cluster(array=w808) -> (cluster=w807:T14)
                    n732 = property on="dig_bits8" class="Clust (strict)"("Value"=w807) -> ()  [unwired: 2 in, 2 out]
                  }
                  frame True {
                    n733 = Array To Cluster(array=w810) -> (cluster=w809:T15)
                    n734 = property on="dig_bits 16" class="Clust (strict)"("Value"=w809) -> ()  [unwired: 2 in, 2 out]
                  }
                }
              }
              frame #4 {
                n735 = local read "Auto-Write"() -> (w815:bool)
                n736 = case shown="True" w815 {
                  frame False {
                  }
                  frame True {
                    n737 = stacked-sequence {
                      frame #0 {
                        n738 = property on="Status" class="Str"("Visible"=FALSE ("Front Panel Window:Resizeable")) -> ()  [unwired: 2 in, 2 out]
                        n739 = property on="Progress" class="Slide (strict)"("Visible"=TRUE ("Front Panel Window:Resizeable")) -> ()  [unwired: 2 in, 2 out]
                      }
                      frame #1 {
                        # "Call external \"Write All Reg\" VI"
                        n740 = local read "Write I2C Address"() -> (w819:u8)
                        n741 = local read "USB DAQ Address"() -> (w821:i32)
                        n742 = local read "Edited Register"() -> (w824:bool[])
                        n743 = control-ref of="Progress"() -> (w822:refnum<vi>)
                        n744 = local read "Register"() -> (w823:u16[])
                        n745 = local read "Index to Reg No"() -> (w818:u8[])
                        n746 = call "Write_All_Reg.vi"("USB DAQ Address"=w821, "Write I2C Address"=w819, "Edited Register"=w824, "Slide Refnum"=w822, "Index to Reg No"=w818, "Register"=w823) -> ("Status"=w820:string)
                        n747 = property on="Status" class="Str"("Val(Sgnl)"=w820) -> ()  [unwired: 2 in, 2 out]
                      }
                      frame #2 {
                        # "Change status of registers to indicate that they have been written to"
                        n748 = local read "Number of Registers"() -> (w828:i32)
                        n749 = local write "Pending changes \nneed to be written"(FALSE ("Pending changes \nneed to be written")) -> ()
                        n750 = Initialize Array(FALSE ("Boolean"), w828) -> (w826:bool[])
                        n751 = local write "Edited Register"(w826) -> ()
                      }
                      frame #3 {
                        # "Remove all bold from table"
                        n752 = local read "Number of Registers"() -> (w829:i32)
                        n753 = for {
                          N: w829 -> [_]
                          i -> [w830]
                          n754 = for {
                            N: 4 -> [_]
                            tunnel: w830 -> [w832]
                            i -> [w833]
                            n755 = stacked-sequence {
                              tunnel: w833 -> [w837 _]
                              tunnel: w832 -> [w836 _]
                              frame #0 {
                                n756 = property on="Register Table" class="MCListbox (strict)"() -> ("ActiveCell"=w835:T13)  [unwired: 2 in, 2 out]
                                n757 = Bundle By Name(cluster=w835, "Row"=w836, "Column"=w837) -> (w834:T13)
                                n758 = property on="Register Table" class="MCListbox (strict)"("ActiveCell"=w834) -> ()  [unwired: 2 in, 2 out]
                              }
                              frame #1 {
                                n759 = property on="Register Table" class="MCListbox (strict)"("CellFontBold"=FALSE ("Active Cell:Cell Font:Bold")) -> ()  [unwired: 2 in, 2 out]
                              }
                            }
                          }
                        }
                      }
                      frame #4 {
                        n760 = property on="Status" class="Str"("Visible"=TRUE ("Front Panel Window:Resizeable")) -> ()  [unwired: 2 in, 2 out]
                        n761 = property on="Progress" class="Slide (strict)"("Visible"=FALSE ("Front Panel Window:Resizeable")) -> ()  [unwired: 2 in, 2 out]
                      }
                    }
                  }
                }
              }
            }
          }
          event "Calculate": Value Change {
            n762 = event-data() -> ()  [unwired: 1 in, 6 out]
            n763 = local read "Enter Current LSB"() -> (w846:dbl)
            "Current LSB" <- w846
            n764 = local read "Shunt Voltage"() -> (w844:dbl)
            "Shunt Voltage" <- w844
            n765 = local read "Current"() -> (w849:dbl)
            "Current" <- w849
            n766 = local read "Power"() -> (w847:dbl)
            "Power" <- w847
            n767 = Divide(x=w844, y=2.5e-06) -> (x/y=→"Shunt Voltage Bin":dbl)
            n768 = Multiply(x=w846, y=25.0) -> (x*y=w848:dbl)
            n769 = Divide(x=w847, y=w848) -> (x/y=→"Power Bin":dbl)
            n770 = Divide(x=w849, y=w846) -> (x/y=→"Current Bin":dbl)
            n771 = local read "Enter Value for \nCalibration Register"() -> (→"Calibration":u16)
            n772 = local read "Enter Rshunt \nVariables"() -> (w855:cluster{"Max Current":dbl, "Resistance":dbl})
            n773 = local read "Bus Voltage"() -> (w843:dbl)
            "Bus Voltage" <- w843
            n774 = Unbundle By Name(w855) -> ("Resistance"=→"Rshunt (Ohms)":dbl)  [unwired: 1 out]
            n775 = Divide(x=w843, y=0.00125) -> (x/y=→"Bus Voltage Bin":dbl)
          }
          event "Enter Rshunt \nVariables": Value Change {
            n776 = event-data() -> ()  [unwired: 1 in, 6 out]
            n777 = local read "Enter Rshunt \nVariables"() -> (w862:cluster{"Max Current":dbl, "Resistance":dbl})
            n778 = Unbundle(w862) -> ("Max Current"=w859:dbl)  [unwired: 1 out]
            n779 = Divide(x=w859, y=u16 4096) -> (x/y=→"High LSB":dbl)
            n780 = Divide(x=w859, y=u16 32768) -> (x/y=→"Low LSB":dbl)
          }
          event "Enter Value for \nCalibration Register": Value Change {
            n781 = event-data() -> ()  [unwired: 1 in, 6 out]
            n782 = flat-sequence {
              tunnel: ["Enter Value for \nCalibration Register"] -> w865
              frame #0 {
                w871 = u16 16  # Word Length
                w872 = u16 0  # Bit Number
                w873 = u16 5  # Reg Number
                n783 = local read "Register"() -> (w874:u16[])
                n784 = call "Change_Bits_in_Reg.vi"("Reg Number"=w873, "Bit Number"=w872, "Word Length"=w871, "Bit Word In"="Enter Value for \nCalibration Register", "Reg In"=w874) -> ("Reg Out"=w870:u16[])
                n785 = property on="Register" class="Arr (strict)"("Val(Sgnl)"=w870) -> ()  [unwired: 2 in, 2 out]
              }
              frame #1 {
                w877 = u16 5  # Reg Number
                n786 = local read "Edited Register"() -> (w876:bool[])
                n787 = Replace Array Subset(array=w876, new element=TRUE ("new element/subarray"), index=w877) -> (w875:bool[])
                n788 = property on="Edited Register" class="Arr (strict)"("Val(Sgnl)"=w875) -> ()  [unwired: 2 in, 2 out]
              }
            }
            n789 = local read "Enter Rshunt \nVariables"() -> (w868:cluster{"Max Current":dbl, "Resistance":dbl})
            n790 = Unbundle(w868) -> ("Resistance"=w864:dbl)  [unwired: 1 out]
            n791 = Multiply(x=w865, y=w864) -> (x*y=w867:dbl)
            n792 = Divide(x=0.00512, y=w867) -> (x/y=w863:dbl)
            n793 = local write "Enter Current LSB"(w863) -> ()
          }
          event "Enter Current LSB": Value Change {
            n794 = event-data() -> ()  [unwired: 1 in, 6 out]
            n795 = local read "Enter Rshunt \nVariables"() -> (w881:cluster{"Max Current":dbl, "Resistance":dbl})
            n796 = Unbundle(w881) -> ("Resistance"=w880:dbl)  [unwired: 1 out]
            n797 = Multiply(x="Enter Current LSB", y=w880) -> (x*y=w884:dbl)
            n798 = Divide(x=0.00512, y=w884) -> (x/y=w879:dbl)
            n799 = flat-sequence {
              tunnel: w879 -> [w885]
              frame #0 {
                w888 = u16 16  # Word Length
                w889 = u16 0  # Bit Number
                w890 = u16 5  # Reg Number
                n800 = local read "Register"() -> (w891:u16[])
                n801 = To Unsigned Word Integer(number=w885) -> (unsigned 16bit integer=w886:u16)
                n802 = local write "Enter Value for \nCalibration Register"(w886) -> ()
                n803 = call "Change_Bits_in_Reg.vi"("Reg Number"=w890, "Bit Number"=w889, "Word Length"=w888, "Bit Word In"=w886, "Reg In"=w891) -> ("Reg Out"=w887:u16[])
                n804 = property on="Register" class="Arr (strict)"("Val(Sgnl)"=w887) -> ()  [unwired: 2 in, 2 out]
              }
              frame #1 {
                w894 = u16 5  # Reg Number
                n805 = local read "Edited Register"() -> (w893:bool[])
                n806 = Replace Array Subset(array=w893, new element=TRUE ("new element/subarray"), index=w894) -> (w892:bool[])
                n807 = property on="Edited Register" class="Arr (strict)"("Val(Sgnl)"=w892) -> ()  [unwired: 2 in, 2 out]
              }
            }
          }
          event "Config Method": Value Change {
            n808 = event-data() -> ()  [unwired: 1 in, 6 out]
            n809 = case shown="\"Calibration Register\"" "Config Method" {
              frame "Current LSB", Default {
                n810 = property on="Enter Value for \nCalibration Register" class="DigNum (strict)"("Visible"=FALSE) -> ()  [unwired: 2 in, 2 out]
                n811 = property on="Max Current" class="DigNum (strict)"("Visible"=TRUE) -> ()  [unwired: 2 in, 2 out]
                n812 = property on="Enter Current LSB" class="DigNum (strict)"("Visible"=TRUE) -> ()  [unwired: 2 in, 2 out]
                n813 = property on="Low LSB" class="DigNum (strict)"("Visible"=TRUE) -> ()  [unwired: 2 in, 2 out]
                n814 = property on="High LSB" class="DigNum (strict)"("Visible"=TRUE) -> ()  [unwired: 2 in, 2 out]
                n815 = property on="Resistance" class="DigNum (strict)"() -> ("Top"=w899:i32)  [unwired: 2 in, 2 out]
                n816 = Subtract(x=w899, y=20) -> (x-y=w897:i32)
                n817 = property on="Resistance" class="DigNum (strict)"("Top"=w897) -> ()  [unwired: 2 in, 2 out]
              }
              frame "Calibration Register" {
                n818 = property on="Enter Value for \nCalibration Register" class="DigNum (strict)"("Visible"=TRUE) -> ()  [unwired: 2 in, 2 out]
                n819 = property on="Max Current" class="DigNum (strict)"("Visible"=FALSE) -> ()  [unwired: 2 in, 2 out]
                n820 = property on="Enter Current LSB" class="DigNum (strict)"("Visible"=FALSE) -> ()  [unwired: 2 in, 2 out]
                n821 = property on="Low LSB" class="DigNum (strict)"("Visible"=FALSE) -> ()  [unwired: 2 in, 2 out]
                n822 = property on="High LSB" class="DigNum (strict)"("Visible"=FALSE) -> ()  [unwired: 2 in, 2 out]
                n823 = property on="Resistance" class="DigNum (strict)"() -> ("Top"=w907:i32)  [unwired: 2 in, 2 out]
                n824 = Add(x=w907, y=20) -> (x+y=w905:i32)
                n825 = property on="Resistance" class="DigNum (strict)"("Top"=w905) -> ()  [unwired: 2 in, 2 out]
              }
            }
          }
        }
      }
    }
  }
